vi "MAI-SIM control.vi"() -> ()   [LabVIEW 2021]
uses:
  <vilib>/DAQmx/write.llb/DAQmx Write (Digital Bool 1Line 1Point).vi
  <vilib>/DAQmx/write.llb/DAQmx Write (Analog DBL 1Chan 1Samp).vi
  <vilib>/DAQmx/read.llb/DAQmx Read (Digital Bool 1Line 1Point).vi
  <vilib>/DAQmx/write.llb/DAQmx Write (Analog Wfm 1Chan NSamp).vi
  <vilib>/DAQmx/create/channels.llb/DAQmx Create Channel (DO-Digital Output).vi
  <vilib>/DAQmx/create/channels.llb/DAQmx Create Channel (DI-Digital Input).vi
  <vilib>/Instr/_visa.llb/VISA Configure Serial Port (Instr).vi
  <vilib>/DAQmx/create/channels.llb/DAQmx Create Channel (AO-Voltage-Basic).vi
  <vilib>/DAQmx/miscellaneous.llb/DAQmx Fill In Error Info.vi
  <vilib>/measure/NI_MABase.lvlib
panel:
  out "?":bool=TRUE
  in  "Go live":bool
  in  "stop":bool=TRUE
  in  "Go SIM":bool
  in  "Tab Control":T1(tab)=enum."Voltages"
  in  "Jog Z":bool
  in  "acquire 405":bool
  in  "405 Exp":dbl=150.0
  out "Images needed":dbl=12.0
  in  "5 phases":bool
  in  "Exposure time":dbl=50.0
  in  "interval /s":dbl
  in  "Timepoints":u32=1 min=1 max=1000 step=1
  in  "647":bool
  in  "561":bool
  in  "488":bool
  in  "405":bool
  in  "Steps /um":dbl
  in  "z-slices":dbl=1.0
  in  "acquire 640":bool
  in  "647 Exp":dbl=150.0
  in  "acquire 561":bool=TRUE
  in  "561 Exp":dbl=80.0
  in  "acquire 488":bool
  in  "488 Exp":dbl=40.0
  in  "Live mode":enum32{"Static", "Strobe", "Widefield", "SIM"}(radio)
  in  "Settle time":u32=30
  in  "Optosplit":T2(radio)=enum."rolling SIM"
  out "odd/even indicator":bool=TRUE
  out "Current voltage":dbl=0.95 format="%#_13g"
  in  "Boolean":bool
  in  "Radio Buttons":enum32{"V1", "V2", "V3"}(radio)
  in  "Debug":dbl[](array[numeric])=[0.95, 0.951, 0.952]
  in  "647 voltages":dbl[][](array[numeric])=[[0.95, 2.25, 3.5], [0.951233, 2.25066, 3.50146], [0.952466, 2.25132, 3.50293]]
  in  "561 voltages":dbl[][](array[numeric])=[[0.95, 2.2, 3.5], [0.951, 2.2025, 3.509], [0.952, 2.2056, 3.518]]
  in  "488 voltages":dbl[][](array[numeric])=[[0.95, 2.25, 3.5], [0.95093, 2.25193, 3.50117], [0.95186, 2.25385, 3.50233]]
  in  "405 voltages":dbl[][](array[numeric])=[[1.0, 0.0, 0.0], [0.0, 0.0, 0.0], [0.0, 0.0, 4.0]]
  out "x+y":i32=8
  in  "647 voltages":dbl[][](array[numeric])=[[0.96, 2.2, 3.5], [0.97, 2.2035, 3.5085], [0.975, 2.2045, 3.5118]]
  in  "561 voltages":dbl[][](array[numeric])=[[0.85, 1.91, 3.2], [0.85065, 1.91064, 3.204], [0.85013, 1.91128, 3.208]]
  in  "488 voltages":dbl[][](array[numeric])=[[0.96, 2.2, 3.5], [0.97, 2.2045, 3.51], [0.975, 2.209, 3.52]]
  in  "405 voltages":dbl[][](array[numeric])=[[1.0, 0.0, 0.0], [0.0, 0.0, 0.0], [0.0, 0.0, 4.0]]
  in  "AOTF channel 2":refnum<visa-resource-name>="COM9"
  in  "405 power":dbl(slide)=1.7857142857142856 min=0.0 max=100.0 step=0.05 scale=0.0..100.0
  in  "405 channel":refnum<visa-resource-name>="COM8"
  in  "488 channel":refnum<visa-resource-name>="COM7"
  in  "488 power":dbl(slide)=1.7647058823529411 min=0.0 max=100.0 step=0.05 scale=0.0..100.0
  in  "ASI stage channel":refnum<visa-resource-name>="COM3"
  in  "physical channels":tag="Dev1/ao0"
  in  "expose any":tag="Dev1/port0/line5"
  in  "647 Power":ext(slide)=14.25 scale=0.0..100.0
  in  "405 shutter":tag="Dev1/port0/line8"
  in  "561 shutter":tag="Dev1/port0/line0"
  in  "488 shutter":tag="Dev1/port0/line1"
  in  "Busy in":tag="Dev1/port0/line3"
  in  "Exposure out":tag="Dev1/port0/line2"
  in  "647 channel":refnum<visa-resource-name>="COM5"
  in  "561 power":dbl(slide)=32.142857142857146 min=0.0 max=100.0 step=0.05 scale=0.0..100.0
  in  "Tab Control 2":T3(tab)
  out "Initialisation error":errorcluster
  out "stage error":errorcluster
  out "Camera/galvo error":errorcluster
  out "Laser error":errorcluster
  out "optosplit stage error":errorcluster
  out "resulting string":string="movrel z=0.000000 \r\n"
  out "resulting string 2":string="movrel z=-0.000000 \r\n"
  in  "short delay":dbl=5.0
  in  "long delay":dbl=55.0
  # "Acquire mode"
  # "o"
  # "o"
  # "o"
  # "o"
  # "o"
  # "o"
  # "o"
  # "o"
  # "o"
  # "o"
  # "o"
  # "o"
  # "-60"
  # "0"
  # "60"
  # "-60"
  # "0"
  # "60"
  # "-60"
  # "0"
  # "60"
  # "-60"
  # "0"
  # "60"
  # "0"
  # "2p/3"
  # "4p/3"
  # "o"
  # "o"
  # "o"
  # "o"
  # "o"
  # "o"
  # "o"
  # "o"
  # "o"
  # "o"
  # "o"
  # "o"
  # "-60"
  # "0"
  # "60"
  # "-60"
  # "0"
  # "60"
  # "-60"
  # "0"
  # "60"
  # "-60"
  # "0"
  # "60"
  # "0"
  # "3p/5"
  # "5p/5"
  # "7p/5"
  # "9p/5"
  # "Hardware lines"
  # "Camera lines"
  # "Laser control"
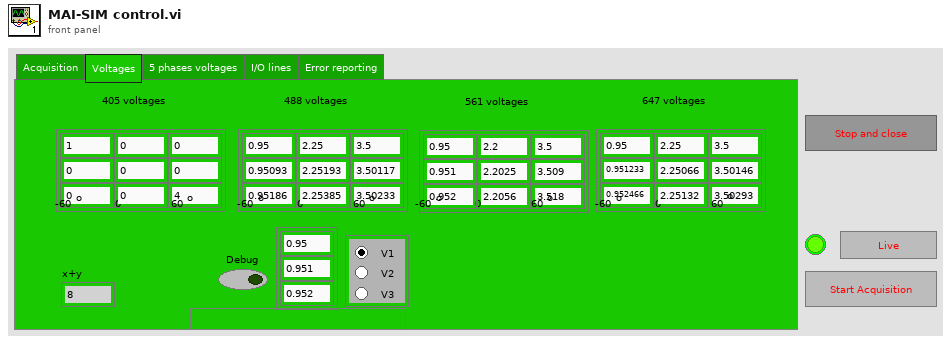
[diagram p1: front panel]
types:
  T1 = enum32{"Acquisition", "Voltages", "5 phases voltages", "I/O lines", "Error reporting"}
  T2 = enum32{"sequential", "optosplit", "fast sequence", "rolling SIM"}
  T3 = enum32{"Page 1", "Page 2", "Page 3", "Page 4", "Page 5"}
  T4 = enum8{"Enabled", "Disabled", "Disabled and Grayed Out"}
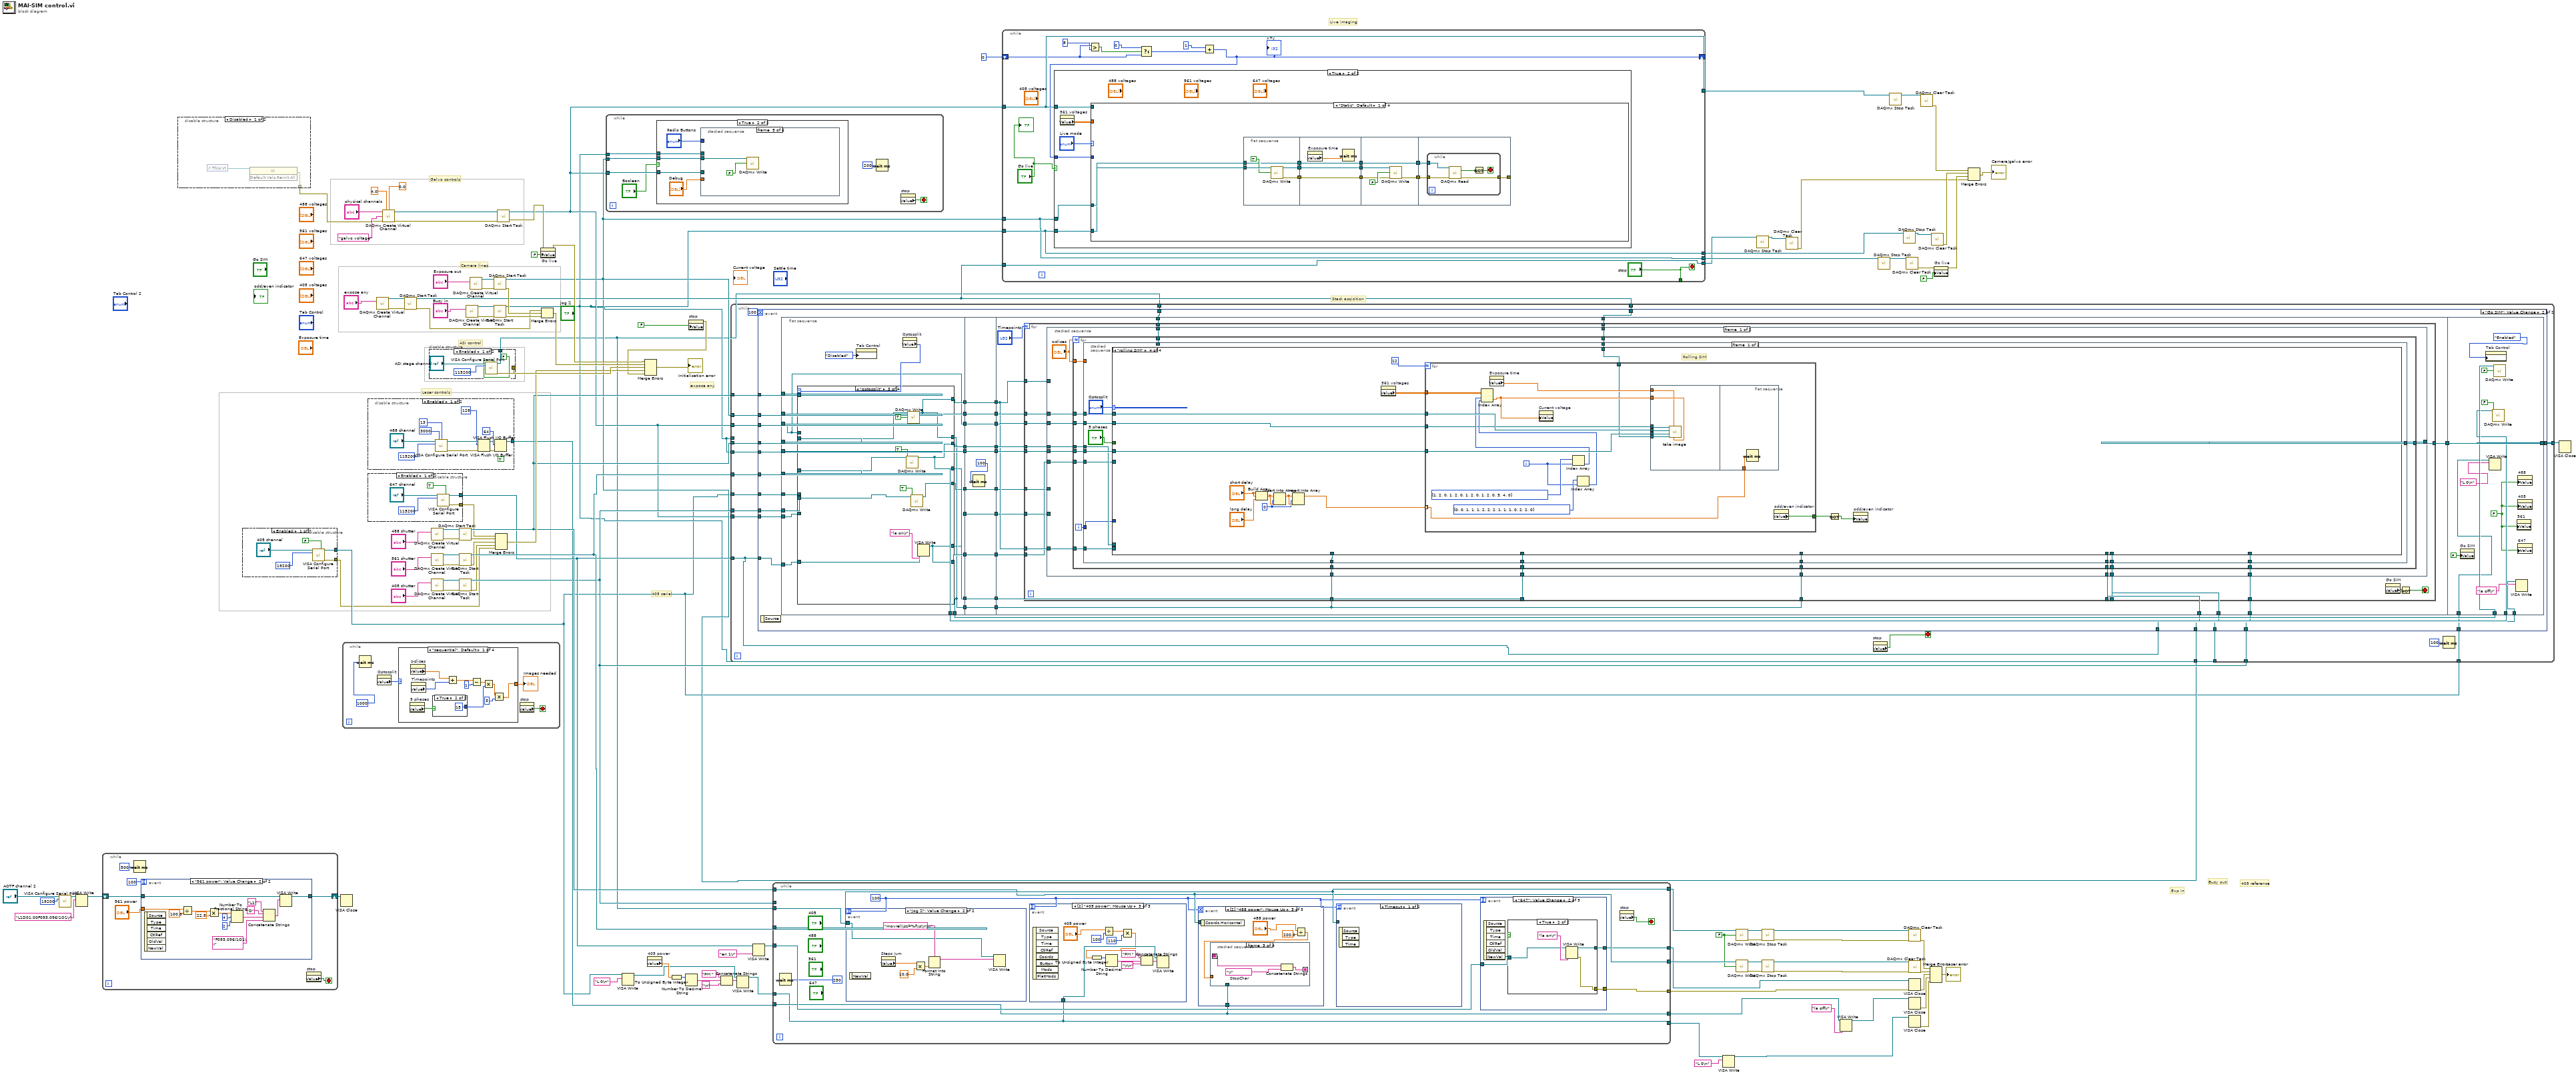
[diagram p0: block diagram]
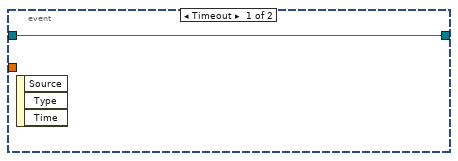
[diagram p2: hidden frame]
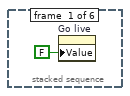
[diagram p7: hidden frame]
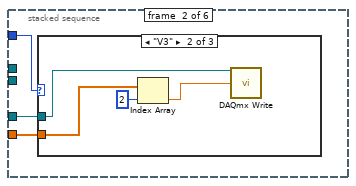
[diagram p8: hidden frame]
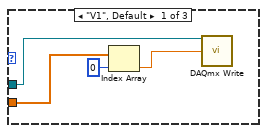
[diagram p9: hidden frame]
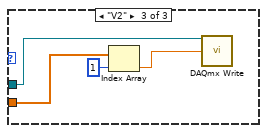
[diagram p10: hidden frame]
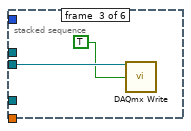
[diagram p11: hidden frame]
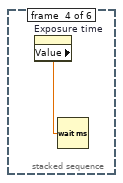
[diagram p12: hidden frame]
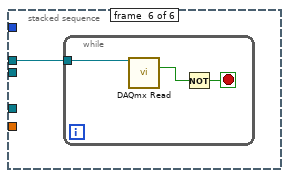
[diagram p13: hidden frame]
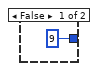
[diagram p15: hidden frame]
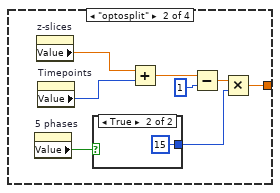
[diagram p16: hidden frame]
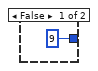
[diagram p17: hidden frame]
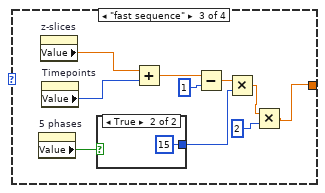
[diagram p18: hidden frame]
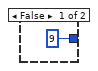
[diagram p19: hidden frame]
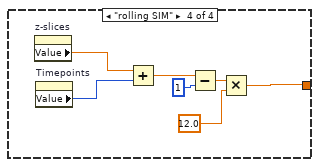
[diagram p20: hidden frame]
diagram:
  w79 = FALSE
  # "405 serial"
  # "expose any"
  # "Busy out"
  # "Exp in"
  # "405 reference"
  # "Stack acqisition"
  # "Live imaging"
  # "Laser controls"
  # "ASI control"
  # "Camera lines"
  # "Galvo controls"
  n1 = call-poly "VISA Configure Serial Port"("VISA resource name"="AOTF channel 2", "baud rate (9600)"=u32 19200) -> ("VISA resource name out"=w2:refnum<visa-resource-name>)  [unwired: 12 in, 1 out]
  n2 = VISA Write(VISA resource name=w2, write buffer="L1D01.00F093.096I1O1\r") -> (VISA resource name out=w1:refnum<visa-resource-name>)  [unwired: 1 in, 2 out]
  n3 = while {
    shift-right: [w116] -> w4
    shift-left: w1 -> [w117]
    stop <- w115 stop-if-true
    n4 = Wait (ms)(milliseconds to wait=500) -> ()  [unwired: 1 out]
    n5 = event shown="[1] \"561 power\": Value Change" {
      selector: _ -> [_ _]
      dyn-events: _ -> [_ _]
      timeout: 100 -> [_ _]
      tunnel: "561 power" -> [_ w132]
      tunnel: w117 -> [w119 w122]
      tunnel: [w119 w121] -> w116
      event Timeout {
        n6 = event-data() -> ()  [unwired: 1 in, 3 out]
      }
      event "561 power": Value Change {
        n7 = event-data() -> ()  [unwired: 1 in, 6 out]
        n8 = Divide(x=w132, y=100.0) -> (x/y=w129:dbl)
        n9 = Multiply(x=w129, y=22.5) -> (x*y=w127:dbl)
        n10 = Number To Fractional String(number=w127, width (-)=4, precision (6)=2) -> (F-format string=w125:string)  [unwired: 1 in]
        n11 = Concatenate Strings("L1", "D", w125, "F093.096I1O1\r") -> (w120:string)
        n12 = VISA Write(VISA resource name=w122, write buffer=w120) -> (VISA resource name out=w121:refnum<visa-resource-name>)  [unwired: 1 in, 2 out]
      }
    }
    n13 = property on="stop" class="Bool (strict)"() -> ("Value"=w115:bool)  [unwired: 2 in, 2 out]
  }
  n14 = disable-structure shown="Disabled" {
    disable-tunnel: [w135 _] -> w26
    frame Disabled {
      n15 = control-ref of="This VI"() -> (w134:refnum<vi>)
      n16 = invoke class="VI" method="Default Vals.Reinit All"(reference=w134) -> (error out=w135:errorcluster)  [unwired: 2 in, 2 out]
    }
    frame Enabled {
    }
  }
  n17 = disable-structure shown="Enabled" {
    disable-tunnel: [w137 _] -> w8
    disable-tunnel: [w136 _] -> w7
    frame Enabled {
      n18 = call-poly "VISA Configure Serial Port"("VISA resource name"="405 channel", "Enable Termination\nChar (T)"=FALSE ("Enable Termination\nChar (T)"), "baud rate (9600)"=u32 19200) -> ("VISA resource name out"=w137:refnum<visa-resource-name>, "error out"=w136:errorcluster)  [unwired: 11 in]
    }
    frame Disabled {
    }
  }
  n19 = VISA Close(VISA resource name=w4) -> ()  [unwired: 1 in, 1 out]
  n20 = while {
    stop <- w143 stop-if-true
    n21 = Wait (ms)(milliseconds to wait=1000) -> ()  [unwired: 1 out]
    n22 = property on="Optosplit" class="RadioBtnsControl (strict)"() -> ("Value"=w142:T2)  [unwired: 2 in, 2 out]
    n23 = case shown="\"sequential\", Default" w142 {
      tunnel: [w145 w162 w167 w180] -> w144
      frame "sequential", Default {
        n24 = property on="5 phases" class="Bool (strict)"() -> ("Value"=w154:bool)  [unwired: 2 in, 2 out]
        n25 = property on="z-slices" class="DigNum (strict)"() -> ("Value"=w152:dbl)  [unwired: 2 in, 2 out]
        n26 = property on="Timepoints" class="DigNum (strict)"() -> ("Value"=w151:u32)  [unwired: 2 in, 2 out]
        n27 = case shown="True" w154 {
          tunnel: [9 15] -> w153
          frame False {
          }
          frame True {
          }
        }
        n28 = Add(x=w152, y=w151) -> (x+y=w149:dbl)
        n29 = Subtract(x=w149, y=1) -> (x-y=w148:dbl)
        n30 = Multiply(x=w148, y=w153) -> (x*y=w147:dbl)
        n31 = Multiply(x=w147, y=3) -> (x*y=w145:dbl)
      }
      frame "optosplit" {
        n32 = property on="5 phases" class="Bool (strict)"() -> ("Value"=w164:bool)  [unwired: 2 in, 2 out]
        n33 = property on="z-slices" class="DigNum (strict)"() -> ("Value"=w161:dbl)  [unwired: 2 in, 2 out]
        n34 = property on="Timepoints" class="DigNum (strict)"() -> ("Value"=w160:u32)  [unwired: 2 in, 2 out]
        n35 = case shown="True" w164 {
          tunnel: [9 15] -> w163
          frame False {
          }
          frame True {
          }
        }
        n36 = Add(x=w161, y=w160) -> (x+y=w158:dbl)
        n37 = Subtract(x=w158, y=1) -> (x-y=w157:dbl)
        n38 = Multiply(x=w157, y=w163) -> (x*y=w162:dbl)
      }
      frame "fast sequence" {
        n39 = property on="5 phases" class="Bool (strict)"() -> ("Value"=w176:bool)  [unwired: 2 in, 2 out]
        n40 = property on="z-slices" class="DigNum (strict)"() -> ("Value"=w174:dbl)  [unwired: 2 in, 2 out]
        n41 = property on="Timepoints" class="DigNum (strict)"() -> ("Value"=w173:u32)  [unwired: 2 in, 2 out]
        n42 = case shown="True" w176 {
          tunnel: [9 15] -> w175
          frame False {
          }
          frame True {
          }
        }
        n43 = Add(x=w174, y=w173) -> (x+y=w171:dbl)
        n44 = Subtract(x=w171, y=1) -> (x-y=w170:dbl)
        n45 = Multiply(x=w170, y=w175) -> (x*y=w169:dbl)
        n46 = Multiply(x=w169, y=2) -> (x*y=w167:dbl)
      }
      frame "rolling SIM" {
        n47 = property on="z-slices" class="DigNum (strict)"() -> ("Value"=w185:dbl)  [unwired: 2 in, 2 out]
        n48 = property on="Timepoints" class="DigNum (strict)"() -> ("Value"=w184:u32)  [unwired: 2 in, 2 out]
        n49 = Add(x=w185, y=w184) -> (x+y=w182:dbl)
        n50 = Subtract(x=w182, y=1) -> (x-y=w181:dbl)
        n51 = Multiply(x=w181, y=12.0) -> (x*y=w180:dbl)
      }
    }
    "Images needed" <- w144
    n52 = property on="stop" class="Bool (strict)"() -> ("Value"=w143:bool)  [unwired: 2 in, 2 out]
  }
  n53 = disable-structure shown="Enabled" {
    disable-tunnel: [w186 _] -> w29
    frame Enabled {
      (unwired) TRUE ("Enable Termination\nChar (T)")
      n54 = call-poly "VISA Configure Serial Port"("VISA resource name"="488 channel", "timeout (10sec)"=u32 3000, "termination char\n(0xA = '\\n' = LF)"=u8 13 ("termination char\n(0xA = '\\n' = LF)"), "baud rate (9600)"=u32 115200) -> ("VISA resource name out"=w196:refnum<visa-resource-name>, "error out"=w195:errorcluster)  [unwired: 5 in, 5 out]
      n55 = VISA Flush I/O Buffer(VISA resource name=w196, mask (16)=u16 128, error in (no error)=w195) -> (VISA resource name out=w192:refnum<visa-resource-name>, error out=w191:errorcluster)
      n56 = VISA Flush I/O Buffer(VISA resource name=w192, mask (16)=u16 64, error in (no error)=w191) -> (VISA resource name out=w186:refnum<visa-resource-name>)  [unwired: 1 out]
    }
    frame Disabled {
    }
  }
  n57 = disable-structure shown="Enabled" {
    disable-tunnel: [w198 _] -> w56
    disable-tunnel: [w197 _] -> w58
    frame Enabled {
      n58 = call-poly "VISA Configure Serial Port"("VISA resource name"="647 channel", "Enable Termination\nChar (T)"=TRUE ("Enable Termination\nChar (T)"), "baud rate (9600)"=u32 115200) -> ("VISA resource name out"=w198:refnum<visa-resource-name>, "error out"=w197:errorcluster)  [unwired: 11 in]
    }
    frame Disabled {
    }
  }
  n59 = call-poly <vilib>:"DAQmx Create Virtual Channel.vi"("lines"="expose any") -> ("task out"=w42:refnum<k21>, "error out"=w41:errorcluster)  [unwired: 13 in]
  n60 = call-poly <vilib>:"DAQmx Create Virtual Channel.vi"("maximum value"=4.0, "minimum value"=0.0, "physical channels"="physical channels", "name to assign"="galvo voltage", "error in"=w26) -> ("task out"=w35:refnum<k21>, "error out"=w34:errorcluster)  [unwired: 9 in]
  n61 = call <vilib>:"DAQmx Start Task.vi"("task/channels in"=w42, "error in"=w41) -> ("task out"=w39:refnum<k21>, "error out"=w40:errorcluster)  [unwired: 12 in]
  n62 = disable-structure shown="Enabled" {
    disable-tunnel: [w204 _] -> w96
    disable-tunnel: [w203 _] -> w25
    frame Enabled {
      n63 = call-poly "VISA Configure Serial Port"("VISA resource name"="ASI stage channel", "Enable Termination\nChar (T)"=FALSE, "baud rate (9600)"=u32 115200) -> ("VISA resource name out"=w203:refnum<visa-resource-name>, "error out"=w204:errorcluster)  [unwired: 11 in]
    }
    frame Disabled {
    }
  }
  n64 = call-poly <vilib>:"DAQmx Create Virtual Channel.vi"("lines"="488 shutter") -> ("task out"=w107:refnum<k21>, "error out"=w108:errorcluster)  [unwired: 13 in]
  n65 = call-poly <vilib>:"DAQmx Create Virtual Channel.vi"("lines"="561 shutter") -> ("task out"=w105:refnum<k21>, "error out"=w106:errorcluster)  [unwired: 13 in]
  n66 = call-poly <vilib>:"DAQmx Create Virtual Channel.vi"("lines"="405 shutter") -> ("task out"=w62:refnum<k21>, "error out"=w63:errorcluster)  [unwired: 13 in]
  n67 = call <vilib>:"DAQmx Start Task.vi"("task/channels in"=w107, "error in"=w108) -> ("task out"=w91:refnum<k21>, "error out"=w100:errorcluster)  [unwired: 12 in]
  n68 = call <vilib>:"DAQmx Start Task.vi"("task/channels in"=w105, "error in"=w106) -> ("task out"=w92:refnum<k21>, "error out"=w99:errorcluster)  [unwired: 12 in]
  n69 = call <vilib>:"DAQmx Start Task.vi"("task/channels in"=w62, "error in"=w63) -> ("task out"=w54:refnum<k21>, "error out"=w30:errorcluster)  [unwired: 12 in]
  n70 = call-poly <vilib>:"DAQmx Create Virtual Channel.vi"("lines"="Busy in") -> ("task out"=w109:refnum<k21>, "error out"=w110:errorcluster)  [unwired: 13 in]
  n71 = call-poly <vilib>:"DAQmx Create Virtual Channel.vi"("lines"="Exposure out") -> ("task out"=w112:refnum<k21>, "error out"=w111:errorcluster)  [unwired: 13 in]
  n72 = call <vilib>:"DAQmx Start Task.vi"("task/channels in"=w112, "error in"=w111) -> ("task out"=w32:refnum<k21>, "error out"=w98:errorcluster)  [unwired: 12 in]
  n73 = call <vilib>:"DAQmx Start Task.vi"("task/channels in"=w109, "error in"=w110) -> ("task out"=w27:refnum<k21>, "error out"=w97:errorcluster)  [unwired: 12 in]
  n74 = Merge Errors(w58, w100, w99, w30, w7) -> (w94:errorcluster)
  n75 = call <vilib>:"DAQmx Start Task.vi"("task/channels in"=w35, "error in"=w34) -> ("task out"=w31:refnum<k21>, "error out"=w52:errorcluster)  [unwired: 12 in]
  n76 = property on="Go live" class="Bool (strict)"(error in=w52, "Value"=FALSE) -> (error out=w51:errorcluster)  [unwired: 1 in, 1 out]
  n77 = Merge Errors(w40, w98, w97) -> (w95:errorcluster)
  n78 = while {
    tunnel: w32 -> [w211]
    tunnel: w27 -> [w210]
    tunnel: w31 -> [w209]
    stop <- w212 stop-if-true
    n79 = case shown="True" "Boolean" {
      tunnel: w211 -> [_ w217]
      tunnel: w210 -> [_ w216]
      tunnel: w209 -> [_ w215]
      frame False {
      }
      frame True {
        n80 = stacked-sequence {
          tunnel: w217 -> [_ _ w235 _ w237 _]
          tunnel: w216 -> [_ _ _ _ _ w239]
          tunnel: "Radio Buttons" -> [_ w221 _ _ _ _]
          tunnel: "Debug" -> [_ w220 _ _ _ _]
          tunnel: w215 -> [_ w219 _ _ _ _]
          frame #0 {
            n81 = property on="Go live" class="Bool (strict)"("Value"=FALSE ("Go live")) -> ()  [unwired: 2 in, 2 out]
          }
          frame #1 {
            n82 = case shown="\"V3\"" w221 {
              tunnel: w220 -> [w224 w228 w232]
              tunnel: w219 -> [w225 w229 w233]
              frame "V1", Default {
                n83 = Index Array(array=w224, index=0) -> (element=w223:dbl)
                n84 = call-poly <vilib>:"DAQmx Write.vi"("task/channels in"=w225, "data"=w223) -> ()  [unwired: 11 in, 3 out]
              }
              frame "V3" {
                n85 = Index Array(array=w228, index=2) -> (element=w227:dbl)
                n86 = call-poly <vilib>:"DAQmx Write.vi"("task/channels in"=w229, "data"=w227) -> ()  [unwired: 11 in, 3 out]
              }
              frame "V2" {
                n87 = Index Array(array=w232, index=1) -> (element=w231:dbl)
                n88 = call-poly <vilib>:"DAQmx Write.vi"("task/channels in"=w233, "data"=w231) -> ()  [unwired: 11 in, 3 out]
              }
            }
          }
          frame #2 {
            n89 = call-poly <vilib>:"DAQmx Write.vi"("task/channels in"=w235, "data"=TRUE) -> ()  [unwired: 11 in, 3 out]
          }
          frame #3 {
            n90 = property on="Exposure time" class="DigNum (strict)"() -> ("Value"=w236:dbl)  [unwired: 2 in, 2 out]
            n91 = Wait (ms)(milliseconds to wait=w236) -> ()  [unwired: 1 out]
          }
          frame #4 {
            n92 = call-poly <vilib>:"DAQmx Write.vi"("task/channels in"=w237, "data"=FALSE) -> ()  [unwired: 11 in, 3 out]
          }
          frame #5 {
            n93 = while {
              tunnel: w239 -> [w240]
              stop <- w242 stop-if-true
              n94 = call-poly <vilib>:"DAQmx Read.vi"("task/channels in"=w240) -> ("data"=w241:bool)  [unwired: 12 in, 2 out]
              n95 = Not(x=w241) -> (.not. x?=w242:bool)
            }
          }
        }
      }
    }
    n96 = Wait (ms)(milliseconds to wait=u32 200) -> ()  [unwired: 1 out]
    n97 = property on="stop" class="Bool (strict)"() -> ("Value"=w212:bool)  [unwired: 2 in, 2 out]
  }
  n98 = VISA Write(VISA resource name=w8, write buffer="L 0\n" ("format string")) -> (VISA resource name out=w17:refnum<visa-resource-name>)  [unwired: 1 in, 2 out]
  n99 = property on="405 power" class="Slide (strict)"() -> ("Value"=w18:dbl)  [unwired: 2 in, 2 out]
  n100 = To Unsigned Byte Integer(number=w18) -> (unsigned 8bit integer=w19:u8)
  n101 = Number To Decimal String(number=w19) -> (decimal integer string=w21:string)  [unwired: 1 in]
  n102 = property on="stop" class="Bool (strict)"("Value"=FALSE) -> (error out=w65:errorcluster)  [unwired: 2 in, 1 out]
  n103 = Merge Errors(w51, w95, w96, w94, w65) -> (→"Initialisation error":errorcluster)
  n104 = Concatenate Strings("PM ", w21, "\n") -> (w23:string)
  n105 = while {
    tunnel: w32 -> [w261]
    tunnel: w27 -> [w260]
    tunnel: w31 -> [w259]
    tunnel: w91 -> [w258]
    tunnel: w92 -> [w257]
    tunnel: w91 -> [w256]
    tunnel: w25 -> [w254]
    tunnel: [w253] -> w67
    tunnel: w27 -> [_]
    tunnel: w56 -> [w251]
    tunnel: w54 -> [w252]
    tunnel: w54 -> [w250]
    tunnel: w32 -> [w249]
    tunnel: w27 -> [w248]
    tunnel: w31 -> [w247]
    tunnel: w39 -> [w246]
    tunnel: w8 -> [w244]
    tunnel: w8 -> [w243]
    stop <- w255 stop-if-true
    n106 = event shown="[1] \"Go SIM\": Value Change" {
      selector: _ -> [_ _]
      dyn-events: _ -> [_ _]
      timeout: 100 -> [_ _]
      tunnel: w261 -> [_ w304]
      tunnel: w260 -> [_ w303]
      tunnel: w259 -> [_ w302]
      tunnel: w258 -> [_ w301]
      tunnel: w257 -> [_ w300]
      tunnel: w256 -> [_ w299]
      tunnel: w254 -> [w263 w298]
      tunnel: [w263 w297] -> w253
      tunnel: w251 -> [_ w293]
      tunnel: w252 -> [_ w292]
      tunnel: w251 -> [_ w291]
      tunnel: w250 -> [_ w290]
      tunnel: w249 -> [_ w289]
      tunnel: w248 -> [_ w288]
      tunnel: w247 -> [_ w287]
      tunnel: w246 -> [_ w266]
      tunnel: w244 -> [_ w265]
      tunnel: w243 -> [_ w264]
      event Timeout {
        n107 = event-data() -> ()  [unwired: 1 in, 3 out]
      }
      event "Go SIM": Value Change {
        n108 = event-data() -> ()  [unwired: 1 in, 1 out]
        n109 = flat-sequence {
          tunnel: [w323] -> w286
          tunnel: w304 -> [w323]
          tunnel: [w322] -> w284
          tunnel: w303 -> [w322]
          tunnel: [w307] -> w282
          tunnel: w302 -> [w307]
          tunnel: w301 -> [w320]
          tunnel: w300 -> [w319]
          tunnel: w299 -> [w318]
          tunnel: [w317] -> w280
          tunnel: [w316] -> w278
          tunnel: [w312] -> w294
          tunnel: [w311] -> w295
          tunnel: w293 -> [w315]
          tunnel: w292 -> [w314]
          tunnel: [w313] -> w276
          tunnel: [w312] -> w274
          tunnel: [w311] -> w272
          tunnel: w287 -> [w310]
          tunnel: [w309] -> w269
          tunnel: [w308] -> w267
          tunnel: w265 -> [w305]
          tunnel: w286 -> [w417]
          tunnel: [w417] -> w285
          tunnel: w284 -> [w416]
          tunnel: [w416] -> w283
          tunnel: w282 -> [w415]
          tunnel: [w415] -> w281
          tunnel: w280 -> [w414]
          tunnel: [w414] -> w279
          tunnel: w278 -> [w413]
          tunnel: [w413] -> w277
          tunnel: w276 -> [w412]
          tunnel: [w412] -> w275
          tunnel: w274 -> [w411]
          tunnel: [w411] -> w273
          tunnel: w272 -> [w410]
          tunnel: [w410] -> w271
          tunnel: [w408] -> w270
          tunnel: w269 -> [w408]
          tunnel: [w407] -> w268
          tunnel: w267 -> [w407]
          tunnel: w285 -> [w434]
          tunnel: w283 -> [w433]
          tunnel: w281 -> [w432]
          tunnel: w279 -> [w431]
          tunnel: w277 -> [w422]
          tunnel: w298 -> [w430]
          tunnel: [w429] -> w296
          tunnel: w275 -> [w428]
          tunnel: w273 -> [w426]
          tunnel: w271 -> [w427]
          tunnel: w290 -> [w425]
          tunnel: w289 -> [w424]
          tunnel: w288 -> [w423]
          tunnel: w270 -> [w421]
          tunnel: w268 -> [w420]
          tunnel: w266 -> [w419]
          tunnel: [w1232] -> w297
          tunnel: w296 -> [w1232]
          tunnel: w295 -> [w1228]
          tunnel: w294 -> [w1229]
          tunnel: w291 -> [w1226]
          tunnel: w264 -> [w1222]
          frame #0 {
            n110 = property on="Tab Control" class="TabCtl (strict)"("DisabledEnum"=T4."Disabled" ("Disabled")) -> ()  [unwired: 2 in, 2 out]
            n111 = property on="Optosplit" class="RadioBtnsControl (strict)"() -> ("Value"=w321:T2)  [unwired: 2 in, 2 out]
            n112 = case shown="\"optosplit\"" w321 {
              tunnel: w320 -> [_ _ _ _]
              tunnel: w319 -> [w334 w356 w375 w394]
              tunnel: w318 -> [w335 w357 w377 w396]
              tunnel: [w333 w355 w374 w393] -> w317
              tunnel: [w332 w354 w376 w395] -> w316
              tunnel: [w333 w355 w374 w393] -> w311
              tunnel: [w332 w354 w376 w395] -> w312
              tunnel: w315 -> [w327 w349 w372 w392]
              tunnel: w314 -> [w330 w352 w370 w382]
              tunnel: [w324 w346 w368 w391] -> w313
              tunnel: [w328 w350 w369 w382] -> w309
              tunnel: w310 -> [w325 w348 _ _]
              tunnel: [w324 w346 w368 w391] -> w308
              tunnel: w307 -> [_ _ _ w383]
              tunnel: w305 -> [_ _ _ w380]
              frame "sequential", Default {
                n113 = property on="odd/even indicator" class="Bool (strict)"() -> ("Value"=w326:bool)  [unwired: 2 in, 2 out]
                n114 = case shown="True" w326 {
                  tunnel: w325 -> [w341 w345]
                  frame False {
                    w339 = 2
                    n115 = property on="647 voltages" class="Arr (strict)"() -> ("Value"=w340:dbl[][])  [unwired: 2 in, 2 out]
                    n116 = Index Array(array=w340, index (row)=w339, index (col)=w339) -> (element=w338:dbl)
                    n117 = call-poly <vilib>:"DAQmx Write.vi"("task/channels in"=w341, "data"=w338) -> ()  [unwired: 11 in, 3 out]
                  }
                  frame True {
                    w343 = 0
                    n118 = property on="561 voltages" class="Arr (strict)"() -> ("Value"=w344:dbl[][])  [unwired: 2 in, 2 out]
                    n119 = Index Array(array=w344, index (row)=w343, index (col)=w343) -> (element=w342:dbl)
                    n120 = call-poly <vilib>:"DAQmx Write.vi"("task/channels in"=w345, "data"=w342) -> ()  [unwired: 11 in, 3 out]
                  }
                }
                n121 = call-poly <vilib>:"DAQmx Write.vi"("task/channels in"=w330, "data"=FALSE) -> ("task out"=w328:refnum<k21>)  [unwired: 11 in, 2 out]
                n122 = call-poly <vilib>:"DAQmx Write.vi"("task/channels in"=w334, "data"=FALSE) -> ("task out"=w333:refnum<k21>)  [unwired: 11 in, 2 out]
                n123 = call-poly <vilib>:"DAQmx Write.vi"("task/channels in"=w335, "data"=FALSE) -> ("task out"=w332:refnum<k21>)  [unwired: 11 in, 2 out]
                n124 = VISA Write(VISA resource name=w327, write buffer="la off\r" ("format string")) -> (VISA resource name out=w324:refnum<visa-resource-name>)  [unwired: 1 in, 2 out]
              }
              frame "fast sequence" {
                n125 = property on="odd/even indicator" class="Bool (strict)"() -> ("Value"=w347:bool)  [unwired: 2 in, 2 out]
                n126 = case shown="True" w347 {
                  tunnel: w348 -> [w363 w367]
                  frame False {
                    w361 = 2
                    n127 = property on="647 voltages" class="Arr (strict)"() -> ("Value"=w362:dbl[][])  [unwired: 2 in, 2 out]
                    n128 = Index Array(array=w362, index (row)=w361, index (col)=w361) -> (element=w360:dbl)
                    n129 = call-poly <vilib>:"DAQmx Write.vi"("task/channels in"=w363, "data"=w360) -> ()  [unwired: 11 in, 3 out]
                  }
                  frame True {
                    w365 = 0
                    n130 = property on="647 voltages" class="Arr (strict)"() -> ("Value"=w366:dbl[][])  [unwired: 2 in, 2 out]
                    n131 = Index Array(array=w366, index (row)=w365, index (col)=w365) -> (element=w364:dbl)
                    n132 = call-poly <vilib>:"DAQmx Write.vi"("task/channels in"=w367, "data"=w364) -> ()  [unwired: 11 in, 3 out]
                  }
                }
                n133 = call-poly <vilib>:"DAQmx Write.vi"("task/channels in"=w352, "data"=FALSE) -> ("task out"=w350:refnum<k21>)  [unwired: 11 in, 2 out]
                n134 = call-poly <vilib>:"DAQmx Write.vi"("task/channels in"=w356, "data"=FALSE) -> ("task out"=w355:refnum<k21>)  [unwired: 11 in, 2 out]
                n135 = call-poly <vilib>:"DAQmx Write.vi"("task/channels in"=w357, "data"=FALSE) -> ("task out"=w354:refnum<k21>)  [unwired: 11 in, 2 out]
                n136 = VISA Write(VISA resource name=w349, write buffer="la off\r" ("format string")) -> (VISA resource name out=w346:refnum<visa-resource-name>)  [unwired: 1 in, 2 out]
              }
              frame "optosplit" {
                n137 = call-poly <vilib>:"DAQmx Write.vi"("task/channels in"=w375, "data"=TRUE) -> ("task out"=w374:refnum<k21>)  [unwired: 11 in, 2 out]
                n138 = call-poly <vilib>:"DAQmx Write.vi"("task/channels in"=w377, "data"=TRUE) -> ("task out"=w376:refnum<k21>)  [unwired: 11 in, 2 out]
                n139 = call-poly <vilib>:"DAQmx Write.vi"("task/channels in"=w370, "data"=TRUE) -> ("task out"=w369:refnum<k21>)  [unwired: 11 in, 2 out]
                n140 = VISA Write(VISA resource name=w372, write buffer="la on\r" ("format string")) -> (VISA resource name out=w368:refnum<visa-resource-name>)  [unwired: 1 in, 2 out]
              }
              frame "rolling SIM" {
                w387 = 0
                n141 = property on="561 voltages" class="Arr (strict)"() -> ("Value"=w388:dbl[][])  [unwired: 2 in, 2 out]
                n142 = property on="acquire 640" class="Bool (strict)"() -> ("Value"=w384:bool)  [unwired: 2 in, 2 out]
                n143 = property on="z-slices" class="DigNum (strict)"("Value"=1) -> ()  [unwired: 2 in, 2 out]
                n144 = property on="acquire 488" class="Bool (strict)"() -> ("Value"=w386:bool)  [unwired: 2 in, 2 out]
                n145 = Index Array(array=w388, index (row)=w387, index (col)=w387) -> (element=w389:dbl)
                n146 = property on="acquire 561" class="Bool (strict)"() -> ("Value"=w385:bool)  [unwired: 2 in, 2 out]
                n147 = property on="acquire 405" class="Bool (strict)"() -> ("Value"=w381:bool)  [unwired: 2 in, 2 out]
                n148 = call-poly <vilib>:"DAQmx Write.vi"("task/channels in"=w383, "data"=w389) -> ()  [unwired: 11 in, 3 out]
                n149 = case shown="False" w381 {
                  tunnel: w380 -> [w397 w399]
                  frame False {
                    n150 = VISA Write(VISA resource name=w397, write buffer="L 0\n" ("format string")) -> ()  [unwired: 1 in, 3 out]
                  }
                  frame True {
                    n151 = VISA Write(VISA resource name=w399, write buffer="L 1\n" ("format string")) -> ()  [unwired: 1 in, 3 out]
                  }
                }
                n152 = case shown="True" w384 {
                  tunnel: w392 -> [w402 w405]
                  tunnel: [w401 w404] -> w391
                  frame False {
                    n153 = VISA Write(VISA resource name=w402, write buffer="la off\r" ("format string")) -> (VISA resource name out=w401:refnum<visa-resource-name>)  [unwired: 1 in, 2 out]
                  }
                  frame True {
                    n154 = VISA Write(VISA resource name=w405, write buffer="la on\r" ("format string")) -> (VISA resource name out=w404:refnum<visa-resource-name>)  [unwired: 1 in, 2 out]
                  }
                }
                n155 = call-poly <vilib>:"DAQmx Write.vi"("task/channels in"=w394, "data"=w385) -> ("task out"=w393:refnum<k21>)  [unwired: 11 in, 2 out]
                n156 = call-poly <vilib>:"DAQmx Write.vi"("task/channels in"=w396, "data"=w386) -> ("task out"=w395:refnum<k21>)  [unwired: 11 in, 2 out]
              }
            }
          }
          frame #1 {
            n157 = Wait (ms)(milliseconds to wait=100) -> ()  [unwired: 1 out]
          }
          frame #2 {
            n158 = for {
              N: "Timepoints" -> [_]
              tunnel: w434 -> [w454]
              tunnel: w433 -> [w453]
              tunnel: w432 -> [w452]
              tunnel: w431 -> [w451]
              tunnel: w422 -> [w450]
              tunnel: w430 -> [w449]
              tunnel: [w448] -> w429
              tunnel: w428 -> [w447]
              tunnel: w427 -> [w446]
              tunnel: w426 -> [w445]
              tunnel: w426 -> [w444]
              tunnel: w425 -> [w443]
              tunnel: w424 -> [w442]
              tunnel: w423 -> [w441]
              tunnel: w422 -> [w440]
              tunnel: w421 -> [w439]
              tunnel: w420 -> [w438]
              tunnel: w419 -> [w437]
              stop <- w435 stop-if-true
              n159 = stacked-sequence {
                tunnel: w454 -> [w470 _]
                tunnel: w453 -> [w469 _]
                tunnel: w452 -> [w468 _]
                tunnel: w451 -> [w467 w1134]
                tunnel: w450 -> [w466 _]
                tunnel: w449 -> [w465 w1136]
                tunnel: [w464 _] -> w448
                tunnel: w447 -> [w463 _]
                tunnel: w446 -> [w462 _]
                tunnel: w445 -> [w461 _]
                tunnel: w444 -> [w460 _]
                tunnel: w443 -> [w459 _]
                tunnel: w442 -> [w458 _]
                tunnel: w441 -> [w457 _]
                tunnel: w440 -> [_ w1135]
                tunnel: w439 -> [_ w1133]
                tunnel: w438 -> [_ w1132]
                tunnel: w437 -> [w455 _]
                frame #0 {
                  n160 = for {
                    N: "z-slices" -> [_]
                    tunnel: w470 -> [w487]
                    tunnel: w469 -> [w486]
                    tunnel: w468 -> [w485]
                    tunnel: w467 -> [w484]
                    tunnel: w466 -> [w483]
                    tunnel: w465 -> [w482]
                    tunnel: [w481] -> w464
                    tunnel: w463 -> [w480]
                    tunnel: w462 -> [w479]
                    tunnel: w461 -> [w478]
                    tunnel: w460 -> [w477]
                    tunnel: w459 -> [w476]
                    tunnel: w458 -> [w475]
                    tunnel: w457 -> [w474]
                    tunnel: "z-slices" -> [w472]
                    tunnel: w455 -> [w471]
                    i -> [w473]
                    n161 = stacked-sequence {
                      tunnel: w487 -> [w502 _]
                      tunnel: w486 -> [w501 _]
                      tunnel: w485 -> [w500 _]
                      tunnel: w484 -> [w499 _]
                      tunnel: w483 -> [w498 _]
                      tunnel: w482 -> [_ w1104]
                      tunnel: [_ w1103] -> w481
                      tunnel: w480 -> [w496 _]
                      tunnel: w479 -> [w495 _]
                      tunnel: w478 -> [w494 _]
                      tunnel: w477 -> [w493 _]
                      tunnel: w476 -> [w492 _]
                      tunnel: w475 -> [w491 _]
                      tunnel: w474 -> [w490 _]
                      tunnel: w473 -> [w489 _]
                      tunnel: w472 -> [_ w1099]
                      tunnel: w471 -> [w488 _]
                      frame #0 {
                        n162 = case shown="\"rolling SIM\"" "Optosplit" {
                          tunnel: w502 -> [w525 w848 w977 w1074]
                          tunnel: w501 -> [w524 w847 w976 w1073]
                          tunnel: w500 -> [w507 w843 w975 w1067]
                          tunnel: w499 -> [w514 _ _ _]
                          tunnel: w498 -> [w513 _ _ _]
                          tunnel: "5 phases" -> [_ _ w974 _]
                          tunnel: w496 -> [w512 w842 _ _]
                          tunnel: w495 -> [w511 w841 _ _]
                          tunnel: w494 -> [w510 _ _ _]
                          tunnel: w493 -> [_ w836 _ _]
                          tunnel: w492 -> [w509 w835 _ _]
                          tunnel: w491 -> [w506 _ _ _]
                          tunnel: w490 -> [w505 _ _ _]
                          tunnel: w489 -> [_ _ _ _]
                          tunnel: w488 -> [w504 w834 w973 w1068]
                          frame "sequential", Default {
                            # "Without optosplit"
                            n163 = case shown="True" "acquire 640" {
                              tunnel: w525 -> [w753 w763]
                              tunnel: w524 -> [w751 w762]
                              tunnel: w507 -> [w752 w756]
                              tunnel: [w753 w760] -> w520
                              tunnel: [w752 w761] -> w521
                              tunnel: [w751 w759] -> w522
                              tunnel: w512 -> [_ w755]
                              tunnel: w504 -> [_ w754]
                              frame False {
                              }
                              frame True {
                                n164 = property on="647 voltages" class="Arr (strict)"() -> ("Value"=w757:dbl[][])  [unwired: 2 in, 2 out]
                                n165 = stacked-sequence {
                                seq-local: [_ w777 _ _] -> [_ _ w797 _]
                                seq-local: [_ w776 _ _] -> [_ _ w796 _]
                                seq-local: [_ w775 _ _] -> [_ _ w795 _]
                                seq-local: [_ w774 _ _] -> [_ _ w791 _]
                                seq-local: [_ w773 _ _] -> [_ _ w790 _]
                                tunnel: w763 -> [_ w777 _ _]
                                tunnel: w756 -> [_ w776 _ _]
                                tunnel: w762 -> [_ w775 _ _]
                                tunnel: w757 -> [_ w774 _ _]
                                tunnel: "647 Exp" -> [_ w773 _ _]
                                tunnel: [_ _ w794 _] -> w761
                                tunnel: [_ _ w793 _] -> w760
                                tunnel: [_ _ w792 _] -> w759
                                tunnel: w757 -> [_ w772 _ _]
                                tunnel: w756 -> [_ w771 _ _]
                                tunnel: w755 -> [w764 _ _ w831]
                                tunnel: w754 -> [_ _ w788 _]
                                frame #0 {
                                n166 = stacked-sequence {
                                tunnel: w764 -> [w765 _]
                                frame #0 {
                                n167 = VISA Write(VISA resource name=w765, write buffer="la on\r" ("format string")) -> ()  [unwired: 1 in, 3 out]
                                }
                                frame #1 {
                                n168 = Wait (ms)(milliseconds to wait=100) -> ()  [unwired: 1 out]
                                }
                                }
                                }
                                frame #1 {
                                n169 = property on="odd/even indicator" class="Bool (strict)"() -> ("Value"=w768:bool)  [unwired: 2 in, 2 out]
                                n170 = case shown="False" w768 {
                                tunnel: [2 0] -> w770
                                tunnel: [2 0] -> w769
                                frame False {
                                }
                                frame True {
                                }
                                }
                                n171 = flat-sequence {
                                tunnel: [w785] -> _
                                tunnel: w772 -> [w787]
                                tunnel: w771 -> [w785]
                                tunnel: [w786] -> _
                                tunnel: w770 -> [w783]
                                tunnel: w769 -> [w782]
                                frame #0 {
                                n172 = Index Array(array=w787, index (row)=w783, index (col)=w782) -> (element=w784:dbl)
                                n173 = call-poly <vilib>:"DAQmx Write.vi"("task/channels in"=w785, "data"=w784) -> ("task out"=w786:refnum<k21>)  [unwired: 11 in, 2 out]
                                }
                                }
                                }
                                frame #2 {
                                n174 = for {
                                N: 9 -> [_]
                                tunnel: w791 -> [w809]
                                tunnel: w797 -> [w806]
                                tunnel: w796 -> [w807]
                                tunnel: w795 -> [w805]
                                tunnel: w790 -> [w808]
                                tunnel: [w807] -> w794
                                tunnel: [w806] -> w793
                                tunnel: [w805] -> w792
                                tunnel: w788 -> [w798]
                                i -> [w801]
                                n175 = property on="odd/even indicator" class="Bool (strict)"() -> ("Value"=w799:bool)  [unwired: 2 in, 2 out]
                                n176 = case shown="True" w799 {
                                tunnel: [i32[] [1, 0, 2, 1, 0, 2, 1, 0, 0, 0, 1, 2, 3, 4, 0] i32[] [1, 2, 0, 1, 2, 0, 1, 2, 2, 0, 1, 2, 3, 4, 0]] -> w804
                                tunnel: [i32[] [2, 2, 1, 1, 1, 0, 0, 0, 0, 2, 2, 2, 2, 2, 0] i32[] [0, 0, 1, 1, 1, 2, 2, 2, 2, 2, 2, 2, 2, 2, 0]] -> w803
                                frame False {
                                }
                                frame True {
                                }
                                }
                                n177 = Index Array(array=w804, index=w801) -> (element=w802:i32)
                                n178 = flat-sequence {
                                tunnel: w809 -> [w818]
                                tunnel: w808 -> [w822]
                                tunnel: w807 -> [w821]
                                tunnel: w806 -> [w820]
                                tunnel: w805 -> [w819]
                                tunnel: w800 -> [w816]
                                tunnel: w802 -> [w815]
                                tunnel: w798 -> [w814]
                                frame #0 {
                                n179 = Index Array(array=w818, index (row)=w815, index (col)=w816) -> (element=w817:dbl)
                                n180 = call "take image.vi"("Voltage"=w817, "Exposure time"=w822, "expose any"=w814, "Busy out"=w819, "Exp In"=w820, "Galvo"=w821) -> ()  [unwired: 6 in]
                                }
                                frame #1 {
                                n181 = property on="Settle time" class="DigNum (strict)"() -> ("Value"=w823:u32)  [unwired: 2 in, 2 out]
                                n182 = Wait (ms)(milliseconds to wait=w823) -> ()  [unwired: 1 out]
                                }
                                }
                                n183 = Index Array(array=w803, index=w801) -> (element=w800:i32)
                                }
                                }
                                frame #3 {
                                n184 = property on="acquire 488" class="Bool (strict)"() -> ("Value"=w827:bool)  [unwired: 2 in, 2 out]
                                n185 = property on="acquire 405" class="Bool (strict)"() -> ("Value"=w826:bool)  [unwired: 2 in, 2 out]
                                n186 = property on="acquire 561" class="Bool (strict)"() -> ("Value"=w828:bool)  [unwired: 2 in, 2 out]
                                n187 = property on="odd/even indicator" class="Bool (strict)"() -> ("Value"=w829:bool)  [unwired: 2 in, 2 out]
                                n188 = Or(x=w828, y=w827) -> (x .or. y?=w825:bool)
                                n189 = Not(x=w829) -> (.not. x?=w830:bool)
                                n190 = Or(x=w825, y=w826) -> (x .or. y?=w824:bool)
                                n191 = case shown="True" w824 {
                                tunnel: w831 -> [_ w832]
                                frame False {
                                }
                                frame True {
                                n192 = VISA Write(VISA resource name=w832, write buffer="la off\r" ("format string")) -> ()  [unwired: 1 in, 3 out]
                                }
                                }
                                n193 = property on="odd/even indicator" class="Bool (strict)"("Value"=w830) -> ()  [unwired: 2 in, 2 out]
                                }
                                }
                              }
                            }
                            n194 = case shown="True" "acquire 561" {
                              tunnel: w522 -> [w670 w681]
                              tunnel: w521 -> [w671 w682]
                              tunnel: [w669 w679] -> w518
                              tunnel: [w671 w680] -> w517
                              tunnel: [w670 w678] -> w516
                              tunnel: w520 -> [w669 w677]
                              tunnel: w514 -> [_ _]
                              tunnel: w507 -> [_ w674]
                              tunnel: w511 -> [_ w673]
                              tunnel: w504 -> [_ w672]
                              frame False {
                              }
                              frame True {
                                n195 = property on="561 voltages" class="Arr (strict)"() -> ("Value"=w675:dbl[][])  [unwired: 2 in, 2 out]
                                n196 = stacked-sequence {
                                seq-local: [_ w692 _ _] -> [_ _ w714 _]
                                seq-local: [_ w691 _ _] -> [_ _ w713 _]
                                seq-local: [_ w690 _ _] -> [_ _ w709 _]
                                seq-local: [_ w689 _ _] -> [_ _ w707 _]
                                seq-local: [_ w688 _ _] -> [_ _ w706 _]
                                tunnel: w682 -> [_ w692 _ _]
                                tunnel: w681 -> [_ w691 _ _]
                                tunnel: w677 -> [_ w690 _ _]
                                tunnel: w675 -> [_ w689 _ _]
                                tunnel: "561 Exp" -> [_ w688 _ _]
                                tunnel: [_ _ w712 _] -> w680
                                tunnel: [_ _ w711 _] -> w679
                                tunnel: [_ _ w710 _] -> w678
                                tunnel: w675 -> [_ w686 _ _]
                                tunnel: w674 -> [_ w685 _ _]
                                tunnel: w673 -> [w684 _ _ w748]
                                tunnel: w672 -> [_ _ w705 _]
                                frame #0 {
                                n197 = call-poly <vilib>:"DAQmx Write.vi"("task/channels in"=w684, "data"=TRUE) -> ()  [unwired: 11 in, 3 out]
                                }
                                frame #1 {
                                n198 = flat-sequence {
                                tunnel: w686 -> [w696]
                                tunnel: [w695] -> w687
                                tunnel: w685 -> [w694]
                                tunnel: [w704] -> _
                                tunnel: w687 -> [w704]
                                frame #0 {
                                n199 = property on="odd/even indicator" class="Bool (strict)"() -> ("Value"=w693:bool)  [unwired: 2 in, 2 out]
                                n200 = case shown="True" w693 {
                                tunnel: [2 0] -> w699
                                tunnel: [2 0] -> w698
                                frame False {
                                }
                                frame True {
                                }
                                }
                                n201 = Index Array(array=w696, index (row)=w699, index (col)=w698) -> (element=w697:dbl)
                                n202 = call-poly <vilib>:"DAQmx Write.vi"("task/channels in"=w694, "data"=w697) -> ("task out"=w695:refnum<k21>)  [unwired: 11 in, 2 out]
                                }
                                frame #1 {
                                }
                                }
                                }
                                frame #2 {
                                n203 = for {
                                N: 9 -> [_]
                                tunnel: w707 -> [w726]
                                tunnel: w709 -> [w723]
                                tunnel: w714 -> [w724]
                                tunnel: w713 -> [w722]
                                tunnel: w706 -> [w725]
                                tunnel: [w724] -> w712
                                tunnel: [w723] -> w711
                                tunnel: [w722] -> w710
                                tunnel: w705 -> [w715]
                                i -> [w719]
                                n204 = property on="odd/even indicator" class="Bool (strict)"() -> ("Value"=w716:bool)  [unwired: 2 in, 2 out]
                                n205 = case shown="False" w716 {
                                tunnel: [i32[] [2, 2, 1, 1, 1, 0, 0, 0, 0, 2, 2, 2, 2, 2, 0] i32[] [0, 0, 1, 1, 1, 2, 2, 2, 2, 2, 2, 2, 2, 2, 0]] -> w721
                                tunnel: [i32[] [1, 0, 2, 1, 0, 2, 1, 0, 0, 0, 1, 2, 3, 4, 0] i32[] [1, 2, 0, 1, 2, 0, 1, 2, 2, 0, 1, 2, 3, 4, 0]] -> w720
                                frame False {
                                }
                                frame True {
                                }
                                }
                                n206 = flat-sequence {
                                tunnel: w726 -> [w735]
                                tunnel: w725 -> [w739]
                                tunnel: w724 -> [w738]
                                tunnel: w723 -> [w737]
                                tunnel: w722 -> [w736]
                                tunnel: w718 -> [w733]
                                tunnel: w717 -> [w732]
                                tunnel: w715 -> [w731]
                                frame #0 {
                                n207 = Index Array(array=w735, index (row)=w733, index (col)=w732) -> (element=w734:dbl)
                                n208 = call "take image.vi"("Voltage"=w734, "Exposure time"=w739, "expose any"=w731, "Busy out"=w736, "Exp In"=w737, "Galvo"=w738) -> ()  [unwired: 6 in]
                                }
                                frame #1 {
                                n209 = property on="Settle time" class="DigNum (strict)"() -> ("Value"=w740:u32)  [unwired: 2 in, 2 out]
                                n210 = Wait (ms)(milliseconds to wait=w740) -> ()  [unwired: 1 out]
                                }
                                }
                                n211 = Index Array(array=w720, index=w719) -> (element=w718:i32)
                                n212 = Index Array(array=w721, index=w719) -> (element=w717:i32)
                                }
                                }
                                frame #3 {
                                n213 = property on="acquire 488" class="Bool (strict)"() -> ("Value"=w744:bool)  [unwired: 2 in, 2 out]
                                n214 = property on="acquire 405" class="Bool (strict)"() -> ("Value"=w745:bool)  [unwired: 2 in, 2 out]
                                n215 = property on="acquire 640" class="Bool (strict)"() -> ("Value"=w743:bool)  [unwired: 2 in, 2 out]
                                n216 = Or(x=w744, y=w745) -> (x .or. y?=w742:bool)
                                n217 = Or(x=w742, y=w743) -> (x .or. y?=w741:bool)
                                n218 = case shown="False" w741 {
                                tunnel: w748 -> [_ w749]
                                frame False {
                                }
                                frame True {
                                n219 = call-poly <vilib>:"DAQmx Write.vi"("task/channels in"=w749, "data"=FALSE) -> ()  [unwired: 11 in, 3 out]
                                }
                                }
                                n220 = property on="odd/even indicator" class="Bool (strict)"() -> ("Value"=w747:bool)  [unwired: 2 in, 2 out]
                                n221 = Not(x=w747) -> (.not. x?=w746:bool)
                                n222 = property on="odd/even indicator" class="Bool (strict)"("Value"=w746) -> ()  [unwired: 2 in, 2 out]
                                }
                                }
                              }
                            }
                            n223 = case shown="True" "acquire 488" {
                              tunnel: w518 -> [w591 w597]
                              tunnel: w516 -> [w589 w601]
                              tunnel: w517 -> [w590 w602]
                              tunnel: [w591 w599] -> _
                              tunnel: [w590 w600] -> _
                              tunnel: [w589 w598] -> _
                              tunnel: w513 -> [_ _]
                              tunnel: w507 -> [_ w594]
                              tunnel: w510 -> [_ w593]
                              tunnel: w504 -> [_ w592]
                              frame False {
                              }
                              frame True {
                                n224 = property on="488 voltages" class="Arr (strict)"() -> ("Value"=w595:dbl[][])  [unwired: 2 in, 2 out]
                                n225 = stacked-sequence {
                                seq-local: [_ w611 _ _] -> [_ _ w632 _]
                                seq-local: [_ w610 _ _] -> [_ _ w631 _]
                                seq-local: [_ w609 _ _] -> [_ _ w627 _]
                                seq-local: [_ w608 _ _] -> [_ _ w625 _]
                                seq-local: [_ w607 _ _] -> [_ _ w624 _]
                                tunnel: w602 -> [_ w611 _ _]
                                tunnel: w601 -> [_ w610 _ _]
                                tunnel: w597 -> [_ w609 _ _]
                                tunnel: w595 -> [_ w608 _ _]
                                tunnel: "488 Exp" -> [_ w607 _ _]
                                tunnel: [_ _ w630 _] -> w600
                                tunnel: [_ _ w629 _] -> w599
                                tunnel: [_ _ w628 _] -> w598
                                tunnel: w595 -> [_ w606 _ _]
                                tunnel: w594 -> [_ w605 _ _]
                                tunnel: w593 -> [w603 _ _ w666]
                                tunnel: w592 -> [_ _ w623 _]
                                frame #0 {
                                n226 = call-poly <vilib>:"DAQmx Write.vi"("task/channels in"=w603, "data"=TRUE) -> ()  [unwired: 11 in, 3 out]
                                }
                                frame #1 {
                                n227 = flat-sequence {
                                tunnel: w606 -> [w618]
                                tunnel: w605 -> [w616]
                                tunnel: [w617] -> _
                                frame #0 {
                                n228 = property on="odd/even indicator" class="Bool (strict)"() -> ("Value"=w612:bool)  [unwired: 2 in, 2 out]
                                n229 = case shown="False" w612 {
                                tunnel: [2 0] -> w614
                                tunnel: [2 0] -> w613
                                frame False {
                                }
                                frame True {
                                }
                                }
                                n230 = Index Array(array=w618, index (row)=w614, index (col)=w613) -> (element=w615:dbl)
                                n231 = call-poly <vilib>:"DAQmx Write.vi"("task/channels in"=w616, "data"=w615) -> ("task out"=w617:refnum<k21>)  [unwired: 11 in, 2 out]
                                }
                                }
                                }
                                frame #2 {
                                n232 = for {
                                N: 9 -> [_]
                                tunnel: w625 -> [w644]
                                tunnel: w627 -> [w642]
                                tunnel: w632 -> [w643]
                                tunnel: w631 -> [w641]
                                tunnel: [w643] -> w630
                                tunnel: [w642] -> w629
                                tunnel: [w641] -> w628
                                tunnel: w624 -> [w640]
                                tunnel: w623 -> [w633]
                                i -> [w639]
                                n233 = property on="odd/even indicator" class="Bool (strict)"() -> ("Value"=w634:bool)  [unwired: 2 in, 2 out]
                                n234 = case shown="True" w634 {
                                tunnel: [i32[] [2, 2, 1, 1, 1, 0, 0, 0, 0, 2, 2, 2, 2, 2, 0] i32[] [0, 0, 1, 1, 1, 2, 2, 2, 2, 2, 2, 2, 2, 2, 0]] -> w635
                                tunnel: [i32[] [1, 0, 2, 1, 0, 2, 1, 0, 0, 0, 1, 2, 3, 4, 0] i32[] [1, 2, 0, 1, 2, 0, 1, 2, 2, 0, 1, 2, 3, 4, 0]] -> w636
                                frame False {
                                }
                                frame True {
                                }
                                }
                                n235 = Index Array(array=w636, index=w639) -> (element=w638:i32)
                                n236 = Index Array(array=w635, index=w639) -> (element=w637:i32)
                                n237 = flat-sequence {
                                tunnel: w644 -> [w653]
                                tunnel: w640 -> [w657]
                                tunnel: w643 -> [w656]
                                tunnel: w642 -> [w655]
                                tunnel: w641 -> [w654]
                                tunnel: w638 -> [w651]
                                tunnel: w637 -> [w650]
                                tunnel: w633 -> [w649]
                                frame #0 {
                                n238 = Index Array(array=w653, index (row)=w651, index (col)=w650) -> (element=w652:dbl)
                                n239 = call "take image.vi"("Voltage"=w652, "Exposure time"=w657, "expose any"=w649, "Busy out"=w654, "Exp In"=w655, "Galvo"=w656) -> ()  [unwired: 6 in]
                                }
                                frame #1 {
                                n240 = property on="Settle time" class="DigNum (strict)"() -> ("Value"=w658:u32)  [unwired: 2 in, 2 out]
                                n241 = Wait (ms)(milliseconds to wait=w658) -> ()  [unwired: 1 out]
                                }
                                }
                                }
                                }
                                frame #3 {
                                n242 = property on="acquire 561" class="Bool (strict)"() -> ("Value"=w662:bool)  [unwired: 2 in, 2 out]
                                n243 = property on="acquire 405" class="Bool (strict)"() -> ("Value"=w661:bool)  [unwired: 2 in, 2 out]
                                n244 = property on="acquire 640" class="Bool (strict)"() -> ("Value"=w663:bool)  [unwired: 2 in, 2 out]
                                n245 = property on="odd/even indicator" class="Bool (strict)"() -> ("Value"=w664:bool)  [unwired: 2 in, 2 out]
                                n246 = Not(x=w664) -> (.not. x?=w665:bool)
                                n247 = Or(x=w662, y=w661) -> (x .or. y?=w660:bool)
                                n248 = property on="odd/even indicator" class="Bool (strict)"("Value"=w665) -> ()  [unwired: 2 in, 2 out]
                                n249 = Or(x=w660, y=w663) -> (x .or. y?=w659:bool)
                                n250 = case shown="True" w659 {
                                tunnel: w666 -> [_ w667]
                                frame False {
                                }
                                frame True {
                                n251 = call-poly <vilib>:"DAQmx Write.vi"("task/channels in"=w667, "data"=FALSE) -> ()  [unwired: 11 in, 3 out]
                                }
                                }
                                }
                                }
                              }
                            }
                            n252 = case shown="True" "acquire 405" {
                              tunnel: w509 -> [_ w532]
                              tunnel: w507 -> [_ w530]
                              tunnel: w506 -> [_ w528]
                              tunnel: w505 -> [_ w527]
                              tunnel: w504 -> [_ w526]
                              frame False {
                              }
                              frame True {
                                n253 = property on="405 voltages" class="Arr (strict)"() -> ("Value"=w531:dbl[][])  [unwired: 2 in, 2 out]
                                n254 = stacked-sequence {
                                tunnel: w531 -> [_ w536 w551 _]
                                tunnel: w530 -> [_ w535 w550 _]
                                tunnel: [_ _ _ w586] -> _
                                tunnel: w532 -> [w533 _ _ w586]
                                tunnel: "405 Exp" -> [_ _ w549 _]
                                tunnel: w528 -> [_ _ w548 _]
                                tunnel: w527 -> [_ _ w547 _]
                                tunnel: w526 -> [_ _ w546 _]
                                frame #0 {
                                n255 = call-poly <vilib>:"DAQmx Write.vi"("task/channels in"=w533, "data"=TRUE) -> ()  [unwired: 11 in, 3 out]
                                }
                                frame #1 {
                                n256 = flat-sequence {
                                tunnel: w536 -> [w540]
                                tunnel: [w539] -> w537
                                tunnel: w535 -> [w538]
                                tunnel: [w545] -> _
                                tunnel: w537 -> [w545]
                                frame #0 {
                                n257 = Index Array(array=w540, index (row)=0, index (col)=0) -> (element=w541:dbl)
                                n258 = call-poly <vilib>:"DAQmx Write.vi"("task/channels in"=w538, "data"=w541) -> ("task out"=w539:refnum<k21>)  [unwired: 11 in, 2 out]
                                }
                                frame #1 {
                                n259 = Wait (ms)(milliseconds to wait=50) -> ()  [unwired: 1 out]
                                }
                                }
                                }
                                frame #2 {
                                n260 = for {
                                N: 9 -> [_]
                                tunnel: w551 -> [w562]
                                tunnel: w550 -> [w561]
                                tunnel: w549 -> [w560]
                                tunnel: w548 -> [w559]
                                tunnel: w547 -> [w558]
                                tunnel: w546 -> [w553]
                                i -> [w557]
                                n261 = property on="odd/even indicator" class="Bool (strict)"() -> ("Value"=w554:bool)  [unwired: 2 in, 2 out]
                                n262 = case shown="True" w554 {
                                tunnel: [i32[] [2, 2, 1, 1, 1, 0, 0, 0, 0, 2, 2, 2, 2, 2, 0] i32[] [0, 0, 1, 1, 1, 2, 2, 2, 2, 2, 2, 2, 2, 2, 0]] -> w556
                                tunnel: [i32[] [1, 0, 2, 1, 0, 2, 1, 0, 0, 0, 1, 2, 3, 4, 0] i32[] [1, 2, 0, 1, 2, 0, 1, 2, 2, 0, 1, 2, 3, 4, 0]] -> w555
                                frame False {
                                }
                                frame True {
                                }
                                }
                                n263 = flat-sequence {
                                tunnel: w564 -> [w576]
                                tunnel: w563 -> [w575]
                                tunnel: w562 -> [w574]
                                tunnel: w561 -> [w573]
                                tunnel: w560 -> [w572]
                                tunnel: w559 -> [w571]
                                tunnel: w558 -> [w570]
                                tunnel: w553 -> [w569]
                                frame #0 {
                                n264 = Index Array(array=w574, index (row)=w576, index (col)=w575) -> (element=w577:dbl)
                                n265 = call "take image.vi"("Voltage"=w577, "Exposure time"=w572, "expose any"=w569, "Busy out"=w570, "Exp In"=w571, "Galvo"=w573) -> ()  [unwired: 6 in]
                                }
                                frame #1 {
                                n266 = property on="Settle time" class="DigNum (strict)"() -> ("Value"=w578:u32)  [unwired: 2 in, 2 out]
                                n267 = Wait (ms)(milliseconds to wait=w578) -> ()  [unwired: 1 out]
                                }
                                }
                                n268 = Index Array(array=w555, index=w557) -> (element=w564:i32)
                                n269 = Index Array(array=w556, index=w557) -> (element=w563:i32)
                                }
                                }
                                frame #3 {
                                n270 = property on="acquire 561" class="Bool (strict)"() -> ("Value"=w581:bool)  [unwired: 2 in, 2 out]
                                n271 = property on="acquire 488" class="Bool (strict)"() -> ("Value"=w582:bool)  [unwired: 2 in, 2 out]
                                n272 = property on="acquire 640" class="Bool (strict)"() -> ("Value"=w580:bool)  [unwired: 2 in, 2 out]
                                n273 = Or(x=w581, y=w582) -> (x .or. y?=w583:bool)
                                n274 = property on="odd/even indicator" class="Bool (strict)"() -> ("Value"=w585:bool)  [unwired: 2 in, 2 out]
                                n275 = Or(x=w583, y=w580) -> (x .or. y?=w579:bool)
                                n276 = Not(x=w585) -> (.not. x?=w584:bool)
                                n277 = property on="odd/even indicator" class="Bool (strict)"("Value"=w584) -> ()  [unwired: 2 in, 2 out]
                                n278 = case shown="True" w579 {
                                tunnel: w586 -> [_ w587]
                                frame False {
                                }
                                frame True {
                                n279 = call-poly <vilib>:"DAQmx Write.vi"("task/channels in"=w587, "data"=FALSE) -> ()  [unwired: 11 in, 3 out]
                                }
                                }
                                }
                                }
                              }
                            }
                          }
                          frame "fast sequence" {
                            # "561"
                            # "488"
                            # "fast sequence"
                            n280 = property on="647 Exp" class="DigNum (strict)"() -> ("Value"=w837:dbl)  [unwired: 2 in, 2 out]
                            n281 = property on="647 voltages" class="Arr (strict)"() -> ("Value"=w840:dbl[][])  [unwired: 2 in, 2 out]
                            n282 = stacked-sequence {
                              seq-local: [_ w922 _ _] -> [_ _ w940 _]
                              seq-local: [_ w921 _ _] -> [_ _ w939 _]
                              seq-local: [_ w920 _ _] -> [_ _ w938 _]
                              seq-local: [_ w919 _ _] -> [_ _ w934 _]
                              seq-local: [_ w918 _ _] -> [_ _ w933 _]
                              tunnel: w848 -> [_ w922 _ _]
                              tunnel: w843 -> [_ w921 _ _]
                              tunnel: w847 -> [_ w920 _ _]
                              tunnel: w840 -> [_ w919 _ _]
                              tunnel: w837 -> [_ w918 _ _]
                              tunnel: [_ _ w937 _] -> w845
                              tunnel: [_ _ w936 _] -> w844
                              tunnel: [_ _ w935 _] -> w846
                              tunnel: w840 -> [_ w916 _ _]
                              tunnel: w843 -> [_ w915 _ _]
                              tunnel: w842 -> [w913 _ _ w971]
                              tunnel: w836 -> [w911 _ _ w969]
                              tunnel: w834 -> [_ _ w931 _]
                              frame #0 {
                                n283 = VISA Write(VISA resource name=w913, write buffer="la on\r" ("format string")) -> ()  [unwired: 1 in, 3 out]
                                n284 = call-poly <vilib>:"DAQmx Write.vi"("task/channels in"=w911, "data"=TRUE) -> ()  [unwired: 11 in, 3 out]
                              }
                              frame #1 {
                                n285 = flat-sequence {
                                tunnel: [w923] -> _
                                tunnel: w916 -> [w925]
                                tunnel: [w924] -> w917
                                tunnel: w915 -> [w923]
                                tunnel: [w930] -> _
                                tunnel: w917 -> [w930]
                                frame #0 {
                                n286 = Index Array(array=w925, index (row)=0, index (col)=0) -> (element=w926:dbl)
                                n287 = call-poly <vilib>:"DAQmx Write.vi"("task/channels in"=w923, "data"=w926) -> ("task out"=w924:refnum<k21>)  [unwired: 11 in, 2 out]
                                }
                                frame #1 {
                                n288 = Wait (ms)(milliseconds to wait=50) -> ()  [unwired: 1 out]
                                }
                                }
                              }
                              frame #2 {
                                n289 = for {
                                N: 9 -> [_]
                                tunnel: w934 -> [w952]
                                tunnel: w940 -> [w949]
                                tunnel: w939 -> [w950]
                                tunnel: w938 -> [w948]
                                tunnel: w933 -> [w951]
                                tunnel: [w950] -> w937
                                tunnel: [w949] -> w936
                                tunnel: [w948] -> w935
                                tunnel: w931 -> [w941]
                                i -> [w946]
                                n290 = property on="odd/even indicator" class="Bool (strict)"() -> ("Value"=w944:bool)  [unwired: 2 in, 2 out]
                                n291 = case shown="False" w944 {
                                tunnel: [i32[] [2, 2, 1, 1, 1, 0, 0, 0, 0, 2, 2, 2, 2, 2, 0] i32[] [0, 0, 1, 1, 1, 2, 2, 2, 2, 2, 2, 2, 2, 2, 0]] -> w942
                                tunnel: [i32[] [1, 0, 2, 1, 0, 2, 1, 0, 0, 0, 1, 2, 3, 4, 0] i32[] [1, 2, 0, 1, 2, 0, 1, 2, 2, 0, 1, 2, 3, 4, 0]] -> w943
                                frame False {
                                }
                                frame True {
                                }
                                }
                                n292 = Index Array(array=w943, index=w946) -> (element=w947:i32)
                                n293 = flat-sequence {
                                tunnel: w952 -> [w961]
                                tunnel: w951 -> [w965]
                                tunnel: w950 -> [w964]
                                tunnel: w949 -> [w963]
                                tunnel: w948 -> [w962]
                                tunnel: w945 -> [w959]
                                tunnel: w947 -> [w958]
                                tunnel: w941 -> [w957]
                                frame #0 {
                                n294 = Index Array(array=w961, index (row)=w958, index (col)=w959) -> (element=w960:dbl)
                                n295 = call "take image.vi"("Voltage"=w960, "Exposure time"=w965, "expose any"=w957, "Busy out"=w962, "Exp In"=w963, "Galvo"=w964) -> ()  [unwired: 6 in]
                                }
                                frame #1 {
                                n296 = property on="Settle time" class="DigNum (strict)"() -> ("Value"=w966:u32)  [unwired: 2 in, 2 out]
                                n297 = Wait (ms)(milliseconds to wait=w966) -> ()  [unwired: 1 out]
                                }
                                }
                                n298 = Index Array(array=w942, index=w946) -> (element=w945:i32)
                                }
                              }
                              frame #3 {
                                n299 = property on="odd/even indicator" class="Bool (strict)"() -> ("Value"=w967:bool)  [unwired: 2 in, 2 out]
                                n300 = Not(x=w967) -> (.not. x?=w968:bool)
                                n301 = property on="odd/even indicator" class="Bool (strict)"("Value"=w968) -> ()  [unwired: 2 in, 2 out]
                                n302 = VISA Write(VISA resource name=w971, write buffer="la off\r" ("format string")) -> ()  [unwired: 1 in, 3 out]
                                n303 = call-poly <vilib>:"DAQmx Write.vi"("task/channels in"=w969, "data"=FALSE) -> ()  [unwired: 11 in, 3 out]
                              }
                            }
                            n304 = property on="561 voltages" class="Arr (strict)"() -> ("Value"=w839:dbl[][])  [unwired: 2 in, 2 out]
                            n305 = property on="561 Exp" class="DigNum (strict)"() -> ("Value"=w838:dbl)  [unwired: 2 in, 2 out]
                            n306 = stacked-sequence {
                              seq-local: [_ w860 _ _] -> [_ _ w878 _]
                              seq-local: [_ w859 _ _] -> [_ _ w877 _]
                              seq-local: [_ w858 _ _] -> [_ _ w873 _]
                              seq-local: [_ w857 _ _] -> [_ _ w871 _]
                              seq-local: [_ w856 _ _] -> [_ _ w870 _]
                              tunnel: w845 -> [_ w860 _ _]
                              tunnel: w846 -> [_ w859 _ _]
                              tunnel: w844 -> [_ w858 _ _]
                              tunnel: w839 -> [_ w857 _ _]
                              tunnel: w838 -> [_ w856 _ _]
                              tunnel: [_ _ w876 _] -> _
                              tunnel: [_ _ w875 _] -> _
                              tunnel: [_ _ w874 _] -> _
                              tunnel: w839 -> [_ w854 _ _]
                              tunnel: w843 -> [_ w853 _ _]
                              tunnel: w841 -> [w852 _ _ w909]
                              tunnel: w835 -> [w849 _ _ w907]
                              tunnel: w834 -> [_ _ w869 _]
                              frame #0 {
                                n307 = call-poly <vilib>:"DAQmx Write.vi"("task/channels in"=w852, "data"=TRUE) -> ()  [unwired: 11 in, 3 out]
                                n308 = call-poly <vilib>:"DAQmx Write.vi"("task/channels in"=w849, "data"=TRUE) -> ()  [unwired: 11 in, 3 out]
                              }
                              frame #1 {
                                n309 = flat-sequence {
                                tunnel: w854 -> [w863]
                                tunnel: [w862] -> w855
                                tunnel: w853 -> [w861]
                                tunnel: [w868] -> _
                                tunnel: w855 -> [w868]
                                frame #0 {
                                n310 = Index Array(array=w863, index (row)=0, index (col)=0) -> (element=w864:dbl)
                                n311 = call-poly <vilib>:"DAQmx Write.vi"("task/channels in"=w861, "data"=w864) -> ("task out"=w862:refnum<k21>)  [unwired: 11 in, 2 out]
                                }
                                frame #1 {
                                n312 = Wait (ms)(milliseconds to wait=50) -> ()  [unwired: 1 out]
                                }
                                }
                              }
                              frame #2 {
                                n313 = for {
                                N: 9 -> [_]
                                tunnel: w871 -> [w890]
                                tunnel: w873 -> [w887]
                                tunnel: w878 -> [w888]
                                tunnel: w877 -> [w886]
                                tunnel: w870 -> [w889]
                                tunnel: [w888] -> w876
                                tunnel: [w887] -> w875
                                tunnel: [w886] -> w874
                                tunnel: w869 -> [w879]
                                i -> [w885]
                                n314 = property on="odd/even indicator" class="Bool (strict)"() -> ("Value"=w880:bool)  [unwired: 2 in, 2 out]
                                n315 = case shown="True" w880 {
                                tunnel: [i32[] [2, 2, 1, 1, 1, 0, 0, 0, 0, 2, 2, 2, 2, 2, 0] i32[] [0, 0, 1, 1, 1, 2, 2, 2, 2, 2, 2, 2, 2, 2, 0]] -> w881
                                tunnel: [i32[] [1, 0, 2, 1, 0, 2, 1, 0, 0, 0, 1, 2, 3, 4, 0] i32[] [1, 2, 0, 1, 2, 0, 1, 2, 2, 0, 1, 2, 3, 4, 0]] -> w882
                                frame False {
                                }
                                frame True {
                                }
                                }
                                n316 = Index Array(array=w882, index=w885) -> (element=w884:i32)
                                n317 = Index Array(array=w881, index=w885) -> (element=w883:i32)
                                n318 = flat-sequence {
                                tunnel: w890 -> [w899]
                                tunnel: w889 -> [w903]
                                tunnel: w888 -> [w902]
                                tunnel: w887 -> [w901]
                                tunnel: w886 -> [w900]
                                tunnel: w884 -> [w897]
                                tunnel: w883 -> [w896]
                                tunnel: w879 -> [w895]
                                frame #0 {
                                n319 = Index Array(array=w899, index (row)=w897, index (col)=w896) -> (element=w898:dbl)
                                n320 = call "take image.vi"("Voltage"=w898, "Exposure time"=w903, "expose any"=w895, "Busy out"=w900, "Exp In"=w901, "Galvo"=w902) -> ()  [unwired: 6 in]
                                }
                                frame #1 {
                                n321 = property on="Settle time" class="DigNum (strict)"() -> ("Value"=w904:u32)  [unwired: 2 in, 2 out]
                                n322 = Wait (ms)(milliseconds to wait=w904) -> ()  [unwired: 1 out]
                                }
                                }
                                }
                              }
                              frame #3 {
                                n323 = call-poly <vilib>:"DAQmx Write.vi"("task/channels in"=w909, "data"=FALSE) -> ()  [unwired: 11 in, 3 out]
                                n324 = property on="odd/even indicator" class="Bool (strict)"() -> ("Value"=w906:bool)  [unwired: 2 in, 2 out]
                                n325 = call-poly <vilib>:"DAQmx Write.vi"("task/channels in"=w907, "data"=FALSE) -> ()  [unwired: 11 in, 3 out]
                                n326 = Not(x=w906) -> (.not. x?=w905:bool)
                                n327 = property on="odd/even indicator" class="Bool (strict)"("Value"=w905) -> ()  [unwired: 2 in, 2 out]
                              }
                            }
                          }
                          frame "optosplit" {
                            n328 = case shown="False" w974 {
                              tunnel: w977 -> [w983 w1020]
                              tunnel: w976 -> [w982 w1019]
                              tunnel: w975 -> [w981 w1018]
                              tunnel: w973 -> [_ w1012]
                              frame True {
                                w978 = 15
                                # "With optosplit"
                                n329 = flat-sequence {
                                tunnel: w981 -> [w987]
                                tunnel: w980 -> [w986]
                                tunnel: [w985] -> w984
                                tunnel: [w994] -> w979
                                tunnel: w984 -> [w994]
                                frame #0 {
                                n330 = Index Array(array=w986, index (row)=0, index (col)=0) -> (element=w988:dbl)
                                n331 = call-poly <vilib>:"DAQmx Write.vi"("task/channels in"=w987, "data"=w988) -> ("task out"=w985:refnum<k21>)  [unwired: 11 in, 2 out]
                                }
                                frame #1 {
                                n332 = property on="Settle time" class="DigNum (strict)"() -> ("Value"=w993:u32)  [unwired: 2 in, 2 out]
                                n333 = Add(x=w993, y=20) -> (x+y=w992:u32)
                                n334 = Wait (ms)(milliseconds to wait=w992) -> ()  [unwired: 1 out]
                                }
                                }
                                n335 = property on="561 voltages" class="Arr (strict)"() -> ("Value"=w980:dbl[][])  [unwired: 2 in, 2 out]
                                n336 = for {
                                N: w978 -> [_]
                                tunnel: w980 -> [w1002]
                                tunnel: w983 -> [w1005]
                                tunnel: w982 -> [w1004]
                                tunnel: w979 -> [w1003]
                                tunnel: w978 -> [_]
                                i -> [w998]
                                n337 = property on="Exposure time" class="DigNum (strict)"() -> ("Value"=w1001:dbl)  [unwired: 2 in, 2 out]
                                n338 = Index Array(array=i32[] [1, 2, 3, 4, 0, 1, 2, 3, 4, 0, 1, 2, 3, 4, 0], index=w998) -> (element=w996:i32)
                                n339 = Index Array(array=i32[] [0, 0, 0, 0, 1, 1, 1, 1, 1, 2, 2, 2, 2, 2, 0], index=w998) -> (element=w997:i32)
                                n340 = Index Array(array=w1002, index (row)=w996, index (col)=w997) -> (element=w995:dbl)
                                n341 = property on="Current voltage" class="DigNum (strict)"("Value"=w995) -> ()  [unwired: 2 in, 2 out]
                                n342 = flat-sequence {
                                tunnel: w1005 -> [w1010]
                                tunnel: w1004 -> [w1009]
                                tunnel: w995 -> [w1008]
                                tunnel: w1003 -> [w1007]
                                tunnel: w1001 -> [w1006]
                                frame #0 {
                                n343 = call "take image.vi"("Voltage"=w1008, "Exposure time"=w1006, "Busy out"=w1009, "Exp In"=w1010, "Galvo"=w1007) -> ()  [unwired: 7 in]
                                }
                                frame #1 {
                                n344 = property on="Settle time" class="DigNum (strict)"() -> ("Value"=w1011:u32)  [unwired: 2 in, 2 out]
                                n345 = Wait (ms)(milliseconds to wait=w1011) -> ()  [unwired: 1 out]
                                }
                                }
                                }
                              }
                              frame False {
                                w1015 = 9
                                # "With optosplit"
                                n346 = flat-sequence {
                                tunnel: w1018 -> [w1027]
                                tunnel: w1017 -> [w1026]
                                tunnel: [w1025] -> w1021
                                tunnel: [w1036] -> w1016
                                tunnel: w1021 -> [w1036]
                                frame #0 {
                                n347 = property on="odd/even indicator" class="Bool (strict)"() -> ("Value"=w1024:bool)  [unwired: 2 in, 2 out]
                                n348 = case shown="False" w1024 {
                                tunnel: [2 0] -> w1023
                                tunnel: [2 0] -> w1022
                                frame False {
                                }
                                frame True {
                                }
                                }
                                n349 = Index Array(array=w1026, index (row)=w1023, index (col)=w1022) -> (element=w1028:dbl)
                                n350 = call-poly <vilib>:"DAQmx Write.vi"("task/channels in"=w1027, "data"=w1028) -> ("task out"=w1025:refnum<k21>)  [unwired: 11 in, 2 out]
                                }
                                frame #1 {
                                n351 = property on="Settle time" class="DigNum (strict)"() -> ("Value"=w1035:u32)  [unwired: 2 in, 2 out]
                                n352 = Add(x=w1035, y=20) -> (x+y=w1034:u32)
                                n353 = Wait (ms)(milliseconds to wait=w1034) -> ()  [unwired: 1 out]
                                }
                                }
                                n354 = property on="561 voltages" class="Arr (strict)"() -> ("Value"=w1017:dbl[][])  [unwired: 2 in, 2 out]
                                n355 = for {
                                N: w1015 -> [_]
                                tunnel: w1017 -> [w1046]
                                tunnel: w1020 -> [w1049]
                                tunnel: w1019 -> [w1048]
                                tunnel: w1016 -> [w1047]
                                tunnel: w1015 -> [_]
                                tunnel: [w1038] -> w1013
                                tunnel: w1012 -> [w1037]
                                i -> [w1044]
                                n356 = property on="odd/even indicator" class="Bool (strict)"() -> ("Value"=w1038:bool)  [unwired: 2 in, 2 out]
                                n357 = property on="Exposure time" class="DigNum (strict)"() -> ("Value"=w1045:dbl)  [unwired: 2 in, 2 out]
                                n358 = case shown="False" w1038 {
                                tunnel: [i32[] [2, 2, 1, 1, 1, 0, 0, 0, 0, 2, 2, 2, 2, 2, 0] i32[] [0, 0, 1, 1, 1, 2, 2, 2, 2, 2, 2, 2, 2, 2, 0]] -> w1039
                                tunnel: [i32[] [1, 0, 2, 1, 0, 2, 1, 0, 0, 0, 1, 2, 3, 4, 0] i32[] [1, 2, 0, 1, 2, 0, 1, 2, 2, 0, 1, 2, 3, 4, 0]] -> w1040
                                frame False {
                                }
                                frame True {
                                }
                                }
                                n359 = Index Array(array=w1040, index=w1044) -> (element=w1042:i32)
                                n360 = Index Array(array=w1039, index=w1044) -> (element=w1043:i32)
                                n361 = Index Array(array=w1046, index (row)=w1042, index (col)=w1043) -> (element=w1041:dbl)
                                n362 = property on="Current voltage" class="DigNum (strict)"("Value"=w1041) -> ()  [unwired: 2 in, 2 out]
                                n363 = flat-sequence {
                                tunnel: w1049 -> [w1059]
                                tunnel: w1048 -> [w1058]
                                tunnel: w1041 -> [w1057]
                                tunnel: w1047 -> [w1056]
                                tunnel: w1045 -> [w1055]
                                tunnel: w1037 -> [w1054]
                                frame #0 {
                                n364 = call "take image.vi"("Voltage"=w1057, "Exposure time"=w1055, "expose any"=w1054, "Busy out"=w1058, "Exp In"=w1059, "Galvo"=w1056) -> ()  [unwired: 6 in]
                                }
                                frame #1 {
                                n365 = property on="Settle time" class="DigNum (strict)"() -> ("Value"=w1060:u32)  [unwired: 2 in, 2 out]
                                n366 = Wait (ms)(milliseconds to wait=w1060) -> ()  [unwired: 1 out]
                                }
                                }
                                }
                                n367 = Not(x=w1013) -> (.not. x?=w1014:bool)
                                n368 = property on="odd/even indicator" class="Bool (strict)"("Value"=w1014) -> ()  [unwired: 2 in, 2 out]
                              }
                            }
                          }
                          frame "rolling SIM" {
                            w1064 = 0 ("index")
                            # "Rolling SIM"
                            n369 = Build Array("short delay", "short delay", "long delay") -> (w1065:dbl[])
                            n370 = Insert Into Array(array=w1065, index=w1064, new element=w1065) -> (w1066:dbl[])
                            n371 = Insert Into Array(array=w1066, index=w1064, new element=w1066) -> (w1061:dbl[])
                            n372 = property on="561 voltages" class="Arr (strict)"() -> ("Value"=w1072:dbl[][])  [unwired: 2 in, 2 out]
                            n373 = for {
                              N: 12 -> [_]
                              tunnel: w1072 -> [w1077]
                              tunnel: w1074 -> [w1088]
                              tunnel: w1073 -> [w1087]
                              tunnel: [w1080] -> w1069
                              tunnel: w1068 -> [w1079]
                              tunnel: w1067 -> [w1078]
                              tunnel: w1061 -> [w1075] mode=indexing
                              i -> [w1076]
                              n374 = property on="Exposure time" class="DigNum (strict)"() -> ("Value"=w1086:dbl)  [unwired: 2 in, 2 out]
                              n375 = Index Array(array=i32[] [1, 2, 0, 1, 2, 0, 1, 2, 0, 1, 2, 0, 3, 4, 0], index=w1076) -> (element=w1084:i32)
                              n376 = Index Array(array=i32[] [0, 0, 1, 1, 1, 2, 2, 2, 1, 1, 1, 0, 2, 2, 0], index=w1076) -> (element=w1085:i32)
                              n377 = Index Array(array=w1077, index (row)=w1084, index (col)=w1085) -> (element=w1083:dbl)
                              n378 = property on="Current voltage" class="DigNum (strict)"("Value"=w1083) -> ()  [unwired: 2 in, 2 out]
                              n379 = flat-sequence {
                                tunnel: w1088 -> [w1094]
                                tunnel: w1087 -> [w1090]
                                tunnel: w1083 -> [w1093]
                                tunnel: w1086 -> [w1092]
                                tunnel: w1079 -> [w1091]
                                tunnel: w1078 -> [w1089]
                                tunnel: w1075 -> [w1095]
                                frame #0 {
                                n380 = call "take image.vi"("Voltage"=w1093, "Exposure time"=w1092, "expose any"=w1091, "Busy out"=w1090, "Exp In"=w1094, "Galvo"=w1089) -> ()  [unwired: 6 in]
                                }
                                frame #1 {
                                n381 = Wait (ms)(milliseconds to wait=w1095) -> ()  [unwired: 1 out]
                                }
                              }
                              n382 = property on="odd/even indicator" class="Bool (strict)"() -> ("Value"=w1080:bool)  [unwired: 2 in, 2 out]
                            }
                            n383 = Not(x=w1069) -> (.not. x?=w1070:bool)
                            n384 = property on="odd/even indicator" class="Bool (strict)"("Value"=w1070) -> ()  [unwired: 2 in, 2 out]
                          }
                        }
                      }
                      frame #1 {
                        n385 = Greater?(x=w1099, y=1) -> (0:w1098:bool)
                        n386 = Greater?(x="Steps /um", y=0) -> (0:w1097:bool)
                        n387 = And(x=w1098, y=w1097) -> (x .and. y?=w1096:bool)
                        n388 = case shown="True" w1096 {
                          tunnel: w1104 -> [w1105 w1108]
                          tunnel: [w1105 w1107] -> w1103
                          tunnel: "Steps /um" -> [_ w1106]
                          frame False {
                          }
                          frame True {
                            n389 = flat-sequence {
                              tunnel: w1108 -> [w1116]
                              tunnel: [w1115] -> w1109
                              tunnel: w1106 -> [w1112]
                              tunnel: [w1119] -> w1107
                              tunnel: w1109 -> [w1119]
                              frame #0 {
                                n390 = Multiply(x=w1112, y=10.0) -> (x*y=w1110:dbl)
                                n391 = Format Into String "Format Into String"(format string="movrel\\sz=%f\\s\\r\\n", w1110) -> (resulting string=w1113:string)  [unwired: 2 in, 1 out]
                                "resulting string" <- w1113
                                n392 = VISA Write(VISA resource name=w1116, write buffer=w1113) -> (VISA resource name out=w1115:refnum<visa-resource-name>, error out=→"optosplit stage error":errorcluster)  [unwired: 1 in, 1 out]
                              }
                              frame #1 {
                                n393 = Wait (ms)(milliseconds to wait=20) -> ()  [unwired: 1 out]
                              }
                            }
                          }
                        }
                      }
                    }
                  }
                }
                frame #1 {
                  n394 = flat-sequence {
                    tunnel: w1135 -> [w1145]
                    tunnel: w1134 -> [w1144]
                    tunnel: w1133 -> [w1143]
                    tunnel: w1132 -> [w1142]
                    tunnel: [w1141] -> w1129
                    tunnel: [w1140] -> w1126
                    tunnel: [w1139] -> w1123
                    tunnel: [w1138] -> w1122
                    tunnel: w1136 -> [w1169]
                    tunnel: [w1168] -> w1130
                    tunnel: w1129 -> [w1168]
                    tunnel: [w1167] -> w1127
                    tunnel: w1126 -> [w1167]
                    tunnel: [w1166] -> w1124
                    tunnel: w1123 -> [w1166]
                    tunnel: w1122 -> [w1165]
                    tunnel: [w1165] -> w1120
                    tunnel: [w1183] -> w1131
                    tunnel: w1130 -> [w1183]
                    tunnel: [w1182] -> w1128
                    tunnel: w1127 -> [w1182]
                    tunnel: [w1181] -> w1125
                    tunnel: w1124 -> [w1181]
                    tunnel: [w1180] -> w1121
                    tunnel: w1120 -> [w1180]
                    tunnel: w1131 -> [w1190]
                    tunnel: w1128 -> [w1189]
                    tunnel: w1125 -> [w1188]
                    tunnel: w1121 -> [w1187]
                    frame #0 {
                      n395 = case shown="False" FALSE {
                        tunnel: w1145 -> [w1149 w1157]
                        tunnel: w1144 -> [w1148 w1156]
                        tunnel: w1143 -> [w1147 w1155]
                        tunnel: w1142 -> [w1146 w1154]
                        tunnel: [w1146 w1153] -> w1141
                        tunnel: [w1147 w1152] -> w1140
                        tunnel: [w1148 w1151] -> w1139
                        tunnel: [w1149 w1150] -> w1138
                        frame False {
                        }
                        frame True {
                          n396 = call-poly <vilib>:"DAQmx Write.vi"("task/channels in"=w1156, "data"=FALSE) -> ("task out"=w1151:refnum<k21>)  [unwired: 11 in, 2 out]
                          n397 = call-poly <vilib>:"DAQmx Write.vi"("task/channels in"=w1157, "data"=FALSE) -> ("task out"=w1150:refnum<k21>)  [unwired: 11 in, 2 out]
                          n398 = call-poly <vilib>:"DAQmx Write.vi"("task/channels in"=w1155, "data"=FALSE) -> ("task out"=w1152:refnum<k21>)  [unwired: 11 in, 2 out]
                          n399 = VISA Write(VISA resource name=w1154, write buffer="la off\r" ("format string")) -> (VISA resource name out=w1153:refnum<visa-resource-name>)  [unwired: 1 in, 2 out]
                        }
                      }
                    }
                    frame #1 {
                      n400 = property on="z-slices" class="DigNum (strict)"() -> ("Value"=w1163:dbl)  [unwired: 2 in, 2 out]
                      n401 = property on="Optosplit" class="RadioBtnsControl (strict)" props=["Value"]() -> ()  [unwired: 2 in, 3 out]
                      n402 = Greater?(x=w1163, y=1) -> (0:w1162:bool)
                      n403 = case shown="False" w1162 {
                        tunnel: w1169 -> [_ w1176]
                        frame False {
                        }
                        frame True {
                          n404 = property on="z-slices" class="DigNum (strict)"() -> ("Value"=w1174:dbl)  [unwired: 2 in, 2 out]
                          n405 = property on="Steps /um" class="DigNum (strict)"() -> ("Value"=w1175:dbl)  [unwired: 2 in, 2 out]
                          n406 = Negate(x=w1175) -> (-x=w1173:dbl)
                          n407 = Multiply(x=w1173, y=w1174) -> (x*y=w1172:dbl)
                          n408 = Multiply(x=w1172, y=10.0) -> (x*y=w1170:dbl)
                          n409 = Format Into String "Format Into String"(format string="movrel\\sz=%f\\s\\r\\n", w1170) -> (resulting string=w1178:string)  [unwired: 2 in, 1 out]
                          "resulting string 2" <- w1178
                          n410 = VISA Write(VISA resource name=w1176, write buffer=w1178) -> (error out=→"stage error":errorcluster)  [unwired: 1 in, 2 out]
                        }
                      }
                    }
                    frame #2 {
                      n411 = Multiply(x="interval /s", y=1000.0) -> (x*y=w1186:dbl)
                      n412 = Wait (ms)(milliseconds to wait=w1186) -> ()  [unwired: 1 out]
                    }
                    frame #3 {
                      n413 = property on="Optosplit" class="RadioBtnsControl (strict)"() -> ("Value"=w1191:T2)  [unwired: 2 in, 2 out]
                      n414 = disable-structure shown="Disabled" {
                        disable-tunnel: w1191 -> [w1196 _]
                        disable-tunnel: w1190 -> [w1195 _]
                        disable-tunnel: w1189 -> [w1194 _]
                        disable-tunnel: w1188 -> [w1193 _]
                        disable-tunnel: w1187 -> [w1192 _]
                        frame Disabled {
                          n415 = case shown="\"rolling SIM\"" w1196 {
                            tunnel: w1195 -> [_ w1200 w1208 w1216]
                            tunnel: w1194 -> [_ w1199 w1207 w1215]
                            tunnel: w1193 -> [_ w1198 w1206 w1214]
                            tunnel: w1192 -> [_ w1197 w1205 w1213]
                            frame "sequential", Default {
                            }
                            frame "optosplit" {
                              n416 = call-poly <vilib>:"DAQmx Write.vi"("task/channels in"=w1198, "data"=TRUE) -> ()  [unwired: 11 in, 3 out]
                              n417 = call-poly <vilib>:"DAQmx Write.vi"("task/channels in"=w1197, "data"=TRUE) -> ()  [unwired: 11 in, 3 out]
                              n418 = call-poly <vilib>:"DAQmx Write.vi"("task/channels in"=w1199, "data"=TRUE) -> ()  [unwired: 11 in, 3 out]
                              n419 = VISA Write(VISA resource name=w1200, write buffer="la on\r" ("format string")) -> ()  [unwired: 1 in, 3 out]
                            }
                            frame "rolling SIM" {
                              n420 = call-poly <vilib>:"DAQmx Write.vi"("task/channels in"=w1206, "data"=TRUE) -> ()  [unwired: 11 in, 3 out]
                              n421 = call-poly <vilib>:"DAQmx Write.vi"("task/channels in"=w1205, "data"=TRUE) -> ()  [unwired: 11 in, 3 out]
                              n422 = call-poly <vilib>:"DAQmx Write.vi"("task/channels in"=w1207, "data"=TRUE) -> ()  [unwired: 11 in, 3 out]
                              n423 = VISA Write(VISA resource name=w1208, write buffer="la on\r" ("format string")) -> ()  [unwired: 1 in, 3 out]
                            }
                            frame "fast sequence" {
                              n424 = call-poly <vilib>:"DAQmx Write.vi"("task/channels in"=w1214, "data"=TRUE) -> ()  [unwired: 11 in, 3 out]
                              n425 = call-poly <vilib>:"DAQmx Write.vi"("task/channels in"=w1213, "data"=TRUE) -> ()  [unwired: 11 in, 3 out]
                              n426 = call-poly <vilib>:"DAQmx Write.vi"("task/channels in"=w1215, "data"=TRUE) -> ()  [unwired: 11 in, 3 out]
                              n427 = VISA Write(VISA resource name=w1216, write buffer="la on\r" ("format string")) -> ()  [unwired: 1 in, 3 out]
                            }
                          }
                        }
                        frame Enabled {
                        }
                      }
                    }
                  }
                }
              }
              n428 = property on="Go SIM" class="Bool (strict)"() -> ("Value"=w436:bool)  [unwired: 2 in, 2 out]
              n429 = Not(x=w436) -> (.not. x?=w435:bool)
            }
          }
          frame #3 {
            w1225 = FALSE
            n430 = property on="Go SIM" class="Bool (strict)"("Value"=FALSE ("Go SIM")) -> ()  [unwired: 2 in, 2 out]
            n431 = property on="Tab Control" class="TabCtl (strict)"("DisabledEnum"=T4."Enabled" ("Disabled")) -> ()  [unwired: 2 in, 2 out]
            n432 = VISA Write(VISA resource name=w1222, write buffer="L 0\n" ("format string")) -> ()  [unwired: 1 in, 3 out]
            n433 = call-poly <vilib>:"DAQmx Write.vi"("task/channels in"=w1228, "data"=FALSE) -> ()  [unwired: 11 in, 3 out]
            n434 = call-poly <vilib>:"DAQmx Write.vi"("task/channels in"=w1229, "data"=FALSE) -> ()  [unwired: 11 in, 3 out]
            n435 = VISA Write(VISA resource name=w1226, write buffer="la off\r" ("format string")) -> ()  [unwired: 1 in, 3 out]
            n436 = property on="561" class="Bool (strict)"("Value"=w1225) -> ()  [unwired: 2 in, 2 out]
            n437 = property on="488" class="Bool (strict)"("Value"=w1225) -> ()  [unwired: 2 in, 2 out]
            n438 = property on="405" class="Bool (strict)"("Value"=w1225) -> ()  [unwired: 2 in, 2 out]
            n439 = property on="647" class="Bool (strict)"("Value"=w1225) -> ()  [unwired: 2 in, 2 out]
          }
        }
      }
    }
    n440 = property on="stop" class="Bool (strict)"() -> ("Value"=w255:bool)  [unwired: 2 in, 2 out]
    n441 = Wait (ms)(milliseconds to wait=u32 100) -> ()  [unwired: 1 out]
  }
  n442 = VISA Write(VISA resource name=w17, write buffer=w23) -> (VISA resource name out=w16:refnum<visa-resource-name>)  [unwired: 1 in, 2 out]
  n443 = VISA Write(VISA resource name=w56, write buffer="en 1\r" ("format string")) -> (VISA resource name out=w55:refnum<visa-resource-name>)  [unwired: 1 in, 2 out]
  n444 = while {
    tunnel: w91 -> [w1242]
    tunnel: w92 -> [w1243]
    tunnel: [w1243] -> w81
    tunnel: [w1242] -> w80
    tunnel: w55 -> [w1238]
    tunnel: w54 -> [_]
    tunnel: [w1240] -> w61
    tunnel: [w1239] -> w60
    tunnel: w29 -> [w1236]
    tunnel: [w1236] -> w10
    tunnel: w25 -> [w1234]
    tunnel: w16 -> [w1233]
    tunnel: [w1233] -> w13
    stop <- w1241 stop-if-true
    w1235 = 100
    n445 = Wait (ms)(milliseconds to wait=u32 250) -> ()  [unwired: 1 out]
    n446 = event shown="[1] \"Jog Z\": Value Change" {
      selector: _ -> [_ _]
      dyn-events: _ -> [_ _]
      timeout: w1235 -> [_ _]
      tunnel: w1234 -> [_ w1245]
      event Timeout {
        n447 = event-data() -> ()  [unwired: 1 in, 3 out]
      }
      event "Jog Z": Value Change {
        n448 = event-data() -> ()  [unwired: 1 in, 1 out]
        n449 = property on="Steps /um" class="DigNum (strict)"() -> ("Value"=w1244:dbl)  [unwired: 2 in, 2 out]
        n450 = Multiply(x=w1244, y=10.0) -> (x*y=w1247:dbl)
        n451 = Format Into String(format string="movrel\\sz=%f\\s\\r\\n", w1247) -> (resulting string=w1248:string)  [unwired: 2 in, 1 out]
        n452 = VISA Write(VISA resource name=w1245, write buffer=w1248) -> ()  [unwired: 1 in, 3 out]
      }
    }
    n453 = event shown="[2] \"405 power\": Mouse Up" {
      selector: _ -> [_ _ _]
      dyn-events: _ -> [_ _ _]
      timeout: w1235 -> [_ _ _]
      tunnel: w1233 -> [_ w1296 w1307]
      event Timeout {
        n454 = event-data() -> ()  [unwired: 1 in, 3 out]
      }
      event "405": Value Change {
        n455 = event-data() -> ("NewVal"=w1297:bool)  [unwired: 1 in, 5 out]
        n456 = case shown="False" w1297 {
          tunnel: w1296 -> [w1298 w1301]
          frame False {
            n457 = VISA Write(VISA resource name=w1298, write buffer="L 0\r\n" ("format string")) -> ()  [unwired: 1 in, 3 out]
          }
          frame True {
            n458 = VISA Write(VISA resource name=w1301, write buffer="L 1\r\n" ("format string")) -> ()  [unwired: 1 in, 3 out]
          }
        }
      }
      event "405 power": Mouse Up {
        n459 = event-data() -> ()  [unwired: 1 in, 8 out]
        n460 = Divide(x="405 power", y=100) -> (x/y=w1306:dbl)
        n461 = Multiply(x=w1306, y=110) -> (x*y=w1302:dbl)
        n462 = To Unsigned Byte Integer(number=w1302) -> (unsigned 8bit integer=w1310:u8)
        n463 = Number To Decimal String(number=w1310) -> (decimal integer string=w1311:string)  [unwired: 1 in]
        n464 = Concatenate Strings("PM ", w1311, "\r\n") -> (w1312:string)
        n465 = VISA Write(VISA resource name=w1307, write buffer=w1312) -> ()  [unwired: 1 in, 3 out]
      }
    }
    n466 = event shown="[2] \"488 power\": Mouse Up" {
      selector: _ -> [_ _ _]
      dyn-events: _ -> [_ _ _]
      timeout: w1235 -> [_ _ _]
      tunnel: w1242 -> [_ w1274 _]
      tunnel: w1236 -> [_ _ w1279]
      event Timeout {
        n467 = event-data() -> ()  [unwired: 1 in, 3 out]
      }
      event "488": Value Change {
        n468 = event-data() -> ("NewVal"=w1275:bool)  [unwired: 1 in, 5 out]
        n469 = call-poly <vilib>:"DAQmx Write.vi"("task/channels in"=w1274, "data"=w1275) -> ()  [unwired: 11 in, 3 out]
      }
      event "488 power": Mouse Up {
        n470 = event-data() -> ()  [unwired: 1 in, 1 out]
        n471 = Divide(x="488 power", y=200.0) -> (x/y=w1276:dbl)
        n472 = stacked-sequence {
          seq-local: [w1280 _ _ _] -> [_ _ w1292 _]
          seq-local: [_ _ w1291 _] -> [_ _ _ w1294]
          tunnel: w1276 -> [w1281 _ _ _]
          tunnel: w1279 -> [_ w1286 _ w1295]
          frame #0 {
            w1285 = "p"  # Command
            n473 = Number To Fractional String(use system decimal point (T)=FALSE, number=w1281) -> (F-format string=w1283:string)  [unwired: 2 in]
            n474 = call <vilib>:"Space Constant.vi"() -> ("String"=w1284:string)
            n475 = Concatenate Strings(w1285, w1284, w1283) -> (w1280:string)
          }
          frame #1 {
            n476 = VISA Flush I/O Buffer(VISA resource name=w1286, mask (16)=u16 128) -> (VISA resource name out=w1289:refnum<visa-resource-name>, error out=w1290:errorcluster)  [unwired: 1 in]
            n477 = VISA Flush I/O Buffer(VISA resource name=w1289, mask (16)=u16 64, error in (no error)=w1290) -> ()  [unwired: 2 out]
          }
          frame #2 {
            w1293 = "\r"  # StopChar
            n478 = Concatenate Strings(w1292, w1293) -> (w1291:string)
          }
          frame #3 {
            n479 = VISA Write(VISA resource name=w1295, write buffer=w1294) -> ()  [unwired: 1 in, 3 out]
          }
        }
      }
    }
    n480 = event shown="[0] Timeout" {
      selector: _ -> [_ _]
      dyn-events: _ -> [_ _]
      timeout: w1235 -> [_ _]
      tunnel: w1243 -> [_ w1272]
      event Timeout {
        n481 = event-data() -> ()  [unwired: 1 in, 3 out]
      }
      event "561": Value Change {
        n482 = event-data() -> ("NewVal"=w1273:bool)  [unwired: 1 in, 5 out]
        n483 = call-poly <vilib>:"DAQmx Write.vi"("task/channels in"=w1272, "data"=w1273) -> ()  [unwired: 11 in, 3 out]
      }
    }
    n484 = event shown="[1] \"647\": Value Change" {
      selector: _ -> [_ _ _]
      dyn-events: _ -> [_ _ _]
      timeout: w1235 -> [_ _ _]
      tunnel: w1238 -> [w1250 w1253 w1267]
      tunnel: [_ w1252 w1264] -> w1239
      tunnel: [w1250 w1251 w1265] -> w1240
      event Timeout {
        n485 = event-data() -> ()  [unwired: 1 in, 3 out]
      }
      event "647": Value Change {
        n486 = event-data() -> ("NewVal"=w1254:bool)  [unwired: 1 in, 5 out]
        n487 = case shown="True" w1254 {
          tunnel: w1253 -> [w1256 w1261]
          tunnel: [w1257 w1260] -> w1252
          tunnel: [w1255 w1259] -> w1251
          frame False {
            n488 = VISA Write(VISA resource name=w1256, write buffer="la off\r" ("format string")) -> (VISA resource name out=w1255:refnum<visa-resource-name>, error out=w1257:errorcluster)  [unwired: 1 in, 1 out]
          }
          frame True {
            n489 = VISA Write(VISA resource name=w1261, write buffer="la on\r" ("format string")) -> (VISA resource name out=w1259:refnum<visa-resource-name>, error out=w1260:errorcluster)  [unwired: 1 in, 1 out]
          }
        }
      }
      event "647 Power": Mouse Up {
        n490 = event-data() -> ()  [unwired: 1 in, 1 out]
        n491 = To Unsigned Byte Integer(number="647 Power") -> (unsigned 8bit integer=w1271:u8)
        n492 = Number To Decimal String(number=w1271) -> (decimal integer string=w1269:string)  [unwired: 1 in]
        n493 = Concatenate Strings("ch 1 pow ", w1269, "\r") -> (w1266:string)
        n494 = VISA Write(VISA resource name=w1267, write buffer=w1266) -> (VISA resource name out=w1265:refnum<visa-resource-name>, error out=w1264:errorcluster)  [unwired: 1 in, 1 out]
      }
    }
    n495 = property on="stop" class="Bool (strict)"() -> ("Value"=w1241:bool)  [unwired: 2 in, 2 out]
  }
  n496 = while {
    tunnel: w31 -> [w1323]
    tunnel: w32 -> [w1322]
    tunnel: w27 -> [w1324]
    tunnel: ["stop"] -> _
    tunnel: [w1324] -> w89
    tunnel: [w1323] -> w88
    tunnel: [w1322] -> w90
    shift-right: [w1316] -> _
    shift-left: 0 -> [w1315]
    tunnel: w39 -> [w1313]
    tunnel: [w1313] -> w38
    stop <- "stop" stop-if-true
    n497 = Greater?(x=w1315, y=8) -> (0:w1318:bool)
    n498 = Select(t=0, s=w1318, f=w1315) -> (s? t:f=w1317:i32)
    n499 = Add(x=1, y=w1317) -> (x+y=w1316:i32)
    "x+y" <- w1316
    n500 = case shown="True" "Go live" {
      tunnel: w1324 -> [_ w1331]
      tunnel: w1323 -> [_ w1330]
      tunnel: w1322 -> [_ w1329]
      tunnel: w1316 -> [_ w1326]
      frame False {
      }
      frame True {
        n501 = property on="561 voltages" class="Arr (strict)"() -> ("Value"=w1327:dbl[][])  [unwired: 2 in, 2 out]
        n502 = case shown="\"Static\", Default" "Live mode" {
          tunnel: w1327 -> [_ w1382 w1432 w1470]
          tunnel: w1330 -> [_ w1379 w1418 w1464]
          tunnel: w1329 -> [w1333 w1365 w1420 _]
          tunnel: w1331 -> [w1332 w1366 w1419 _]
          tunnel: w1326 -> [_ _ w1408 _]
          frame "Static", Default {
            n503 = flat-sequence {
              tunnel: w1333 -> [w1346]
              tunnel: [w1344] -> w1341
              tunnel: [w1343] -> w1340
              tunnel: w1332 -> [w1342]
              tunnel: [w1342] -> w1339
              tunnel: w1341 -> [w1350]
              tunnel: [w1350] -> w1338
              tunnel: w1340 -> [w1348]
              tunnel: [w1349] -> w1337
              tunnel: w1339 -> [w1349]
              tunnel: [w1348] -> w1336
              tunnel: w1338 -> [w1355]
              tunnel: [w1353] -> w1335
              tunnel: w1337 -> [w1353]
              tunnel: w1336 -> [w1352]
              tunnel: [w1351] -> w1334
              tunnel: w1335 -> [w1358]
              tunnel: w1334 -> [w1357]
              tunnel: [w1356] -> _
              frame #0 {
                n504 = call-poly <vilib>:"DAQmx Write.vi"("task/channels in"=w1346, "data"=TRUE) -> ("task out"=w1344:refnum<k21>, "error out"=w1343:errorcluster)  [unwired: 11 in, 1 out]
              }
              frame #1 {
                n505 = property on="Exposure time" class="DigNum (strict)"() -> ("Value"=w1347:dbl)  [unwired: 2 in, 2 out]
                n506 = Wait (ms)(milliseconds to wait=w1347) -> ()  [unwired: 1 out]
              }
              frame #2 {
                n507 = call-poly <vilib>:"DAQmx Write.vi"("task/channels in"=w1355, "data"=FALSE, "error in"=w1352) -> ("error out"=w1351:errorcluster)  [unwired: 10 in, 2 out]
              }
              frame #3 {
                n508 = while {
                  tunnel: w1358 -> [w1363]
                  tunnel: w1357 -> [w1362]
                  tunnel: [w1361] -> w1356
                  stop <- w1360 stop-if-true
                  n509 = call-poly <vilib>:"DAQmx Read.vi"("task/channels in"=w1363, "error in"=w1362) -> ("data"=w1359:bool, "error out"=w1361:errorcluster)  [unwired: 11 in, 1 out]
                  n510 = Not(x=w1359) -> (.not. x?=w1360:bool)
                }
              }
            }
          }
          frame "Widefield" {
            n511 = Index Array(array=w1382, index (row)=2, index (col)=1) -> ()  [unwired: 1 out]
            n512 = call <vilib>:"Triangle Waveform.vi"("offset"=1.0, "phase"=0.0, "amplitude"=0.06, "frequency"=0.1) -> ("signal out"=w1375:waveform(dbl))  [unwired: 6 in, 1 out]
            n513 = call-poly <vilib>:"DAQmx Write.vi"("task/channels in"=w1379, "data"=w1375) -> ()  [unwired: 11 in, 3 out]
            n514 = flat-sequence {
              tunnel: w1365 -> [w1387]
              tunnel: [w1385] -> w1374
              tunnel: [w1384] -> w1373
              tunnel: [w1383] -> w1372
              tunnel: w1366 -> [w1383]
              tunnel: w1374 -> [w1391]
              tunnel: [w1391] -> w1371
              tunnel: w1373 -> [w1389]
              tunnel: [w1390] -> w1370
              tunnel: w1372 -> [w1390]
              tunnel: [w1389] -> w1369
              tunnel: w1371 -> [w1396]
              tunnel: [w1394] -> w1368
              tunnel: w1370 -> [w1394]
              tunnel: w1369 -> [w1393]
              tunnel: [w1392] -> w1367
              tunnel: w1368 -> [w1399]
              tunnel: w1367 -> [w1398]
              tunnel: [w1397] -> _
              frame #0 {
                n515 = call-poly <vilib>:"DAQmx Write.vi"("task/channels in"=w1387, "data"=TRUE) -> ("task out"=w1385:refnum<k21>, "error out"=w1384:errorcluster)  [unwired: 11 in, 1 out]
              }
              frame #1 {
                n516 = property on="Exposure time" class="DigNum (strict)"() -> ("Value"=w1388:dbl)  [unwired: 2 in, 2 out]
                n517 = Wait (ms)(milliseconds to wait=w1388) -> ()  [unwired: 1 out]
              }
              frame #2 {
                n518 = call-poly <vilib>:"DAQmx Write.vi"("task/channels in"=w1396, "data"=FALSE, "error in"=w1393) -> ("error out"=w1392:errorcluster)  [unwired: 10 in, 2 out]
              }
              frame #3 {
                n519 = while {
                  tunnel: w1399 -> [w1404]
                  tunnel: w1398 -> [w1403]
                  tunnel: [w1402] -> w1397
                  stop <- w1401 stop-if-true
                  n520 = call-poly <vilib>:"DAQmx Read.vi"("task/channels in"=w1404, "error in"=w1403) -> ("data"=w1400:bool, "error out"=w1402:errorcluster)  [unwired: 11 in, 1 out]
                  n521 = Not(x=w1400) -> (.not. x?=w1401:bool)
                }
              }
            }
          }
          frame "SIM" {
            n522 = Quotient & Remainder(x=w1408, y=9) -> (x-y*floor(x/y)=w1430:i32)  [unwired: 1 out]
            n523 = flat-sequence {
              tunnel: w1419 -> [w1436]
              tunnel: w1420 -> [w1437]
              tunnel: [w1437] -> w1417
              tunnel: [w1433] -> w1415
              tunnel: [w1436] -> w1413
              tunnel: w1418 -> [w1435]
              tunnel: w1407 -> [w1434]
              tunnel: w1417 -> [w1441]
              tunnel: [w1441] -> w1416
              tunnel: w1415 -> [w1440]
              tunnel: [w1440] -> w1414
              tunnel: w1413 -> [w1439]
              tunnel: [w1439] -> w1412
              tunnel: [w1445] -> w1428
              tunnel: [w1443] -> w1427
              tunnel: [w1442] -> w1426
              tunnel: w1416 -> [w1447]
              tunnel: w1414 -> [w1444]
              tunnel: w1412 -> [w1442]
              tunnel: w1428 -> [w1451]
              tunnel: [w1451] -> w1425
              tunnel: w1427 -> [w1449]
              tunnel: [w1450] -> w1424
              tunnel: w1426 -> [w1450]
              tunnel: [w1449] -> w1423
              tunnel: w1425 -> [w1456]
              tunnel: [w1454] -> w1422
              tunnel: w1424 -> [w1454]
              tunnel: w1423 -> [w1453]
              tunnel: [w1452] -> w1421
              tunnel: w1422 -> [w1458]
              tunnel: w1421 -> [w1457]
              frame #0 {
                n524 = call-poly <vilib>:"DAQmx Write.vi"("task/channels in"=w1435, "data"=w1434) -> ("error out"=w1433:errorcluster)  [unwired: 11 in, 2 out]
              }
              frame #1 {
                n525 = property on="Settle time" class="DigNum (strict)"() -> ("Value"=w1438:u32)  [unwired: 2 in, 2 out]
                n526 = Wait (ms)(milliseconds to wait=w1438) -> ()  [unwired: 1 out]
              }
              frame #2 {
                n527 = call-poly <vilib>:"DAQmx Write.vi"("task/channels in"=w1447, "data"=TRUE, "error in"=w1444) -> ("task out"=w1445:refnum<k21>, "error out"=w1443:errorcluster)  [unwired: 10 in, 1 out]
              }
              frame #3 {
                n528 = property on="Exposure time" class="DigNum (strict)"() -> ("Value"=w1448:dbl)  [unwired: 2 in, 2 out]
                n529 = Wait (ms)(milliseconds to wait=w1448) -> ()  [unwired: 1 out]
              }
              frame #4 {
                n530 = call-poly <vilib>:"DAQmx Write.vi"("task/channels in"=w1456, "data"=FALSE, "error in"=w1453) -> ("error out"=w1452:errorcluster)  [unwired: 10 in, 2 out]
              }
              frame #5 {
                n531 = while {
                  tunnel: w1458 -> [w1463]
                  tunnel: w1457 -> [w1462]
                  tunnel: [w1461] -> _
                  stop <- w1460 stop-if-true
                  n532 = call-poly <vilib>:"DAQmx Read.vi"("task/channels in"=w1463, "error in"=w1462) -> ("data"=w1459:bool, "error out"=w1461:errorcluster)  [unwired: 11 in, 1 out]
                  n533 = Not(x=w1459) -> (.not. x?=w1460:bool)
                }
              }
            }
            n534 = Add(x=0, y=w1430) -> (x+y=w1409:i32)
            n535 = Index Array(array=i32[] [1, 2, 0, 1, 2, 0, 1, 2, 0, 0, 1, 2, 3, 4, 0], index=w1409) -> (element=w1405:i32)
            n536 = Index Array(array=i32[] [0, 0, 1, 1, 1, 2, 2, 2, 0, 2, 2, 2, 2, 2, 0], index=w1409) -> (element=w1406:i32)
            n537 = Index Array(array=w1432, index (row)=w1405, index (col)=w1406) -> (element=w1407:dbl)
            n538 = property on="Current voltage" class="DigNum (strict)"("Value"=w1407) -> ()  [unwired: 2 in, 2 out]
          }
          frame "Strobe" {
            n539 = flat-sequence {
              tunnel: w1470 -> [w1472]
              tunnel: [w1472] -> w1468
              tunnel: w1464 -> [w1471]
              tunnel: [w1477] -> w1469
              tunnel: w1468 -> [w1477]
              tunnel: w1469 -> [w1479]
              tunnel: [w1479] -> w1467
              tunnel: w1464 -> [w1478]
              tunnel: w1467 -> [w1484]
              tunnel: [w1484] -> w1466
              tunnel: w1466 -> [w1486]
              tunnel: [w1486] -> w1465
              tunnel: w1464 -> [w1485]
              tunnel: [w1491] -> _
              tunnel: w1465 -> [w1491]
              frame #0 {
                n540 = Index Array(array=w1472, index (row)=2, index (col)=0) -> (element=w1473:dbl)
                n541 = call-poly <vilib>:"DAQmx Write.vi"("task/channels in"=w1471, "data"=w1473) -> ()  [unwired: 11 in, 3 out]
              }
              frame #1 {
                n542 = property on="Settle time" class="DigNum (strict)"() -> ("Value"=w1476:u32)  [unwired: 2 in, 2 out]
                n543 = Wait (ms)(milliseconds to wait=w1476) -> ()  [unwired: 1 out]
              }
              frame #2 {
                n544 = Index Array(array=w1479, index (row)=2, index (col)=1) -> (element=w1482:dbl)
                n545 = call-poly <vilib>:"DAQmx Write.vi"("task/channels in"=w1478, "data"=w1482) -> ()  [unwired: 11 in, 3 out]
              }
              frame #3 {
                n546 = property on="Settle time" class="DigNum (strict)"() -> ("Value"=w1483:u32)  [unwired: 2 in, 2 out]
                n547 = Wait (ms)(milliseconds to wait=w1483) -> ()  [unwired: 1 out]
              }
              frame #4 {
                n548 = Index Array(array=w1486, index (row)=2, index (col)=2) -> (element=w1487:dbl)
                n549 = call-poly <vilib>:"DAQmx Write.vi"("task/channels in"=w1485, "data"=w1487) -> ()  [unwired: 11 in, 3 out]
              }
              frame #5 {
                n550 = property on="Settle time" class="DigNum (strict)"() -> ("Value"=w1490:u32)  [unwired: 2 in, 2 out]
                n551 = Wait (ms)(milliseconds to wait=w1490) -> ()  [unwired: 1 out]
              }
            }
          }
        }
      }
    }
    "?" <- "Go live"
  }
  n552 = VISA Write(VISA resource name=w13, write buffer="L 0\n" ("format string")) -> (VISA resource name out=w12:refnum<visa-resource-name>)  [unwired: 1 in, 2 out]
  n553 = call-poly <vilib>:"DAQmx Write.vi"("task/channels in"=w81, "data"=w79) -> ("task out"=w75:refnum<k21>, "error out"=w73:errorcluster)  [unwired: 11 in, 1 out]
  n554 = call-poly <vilib>:"DAQmx Write.vi"("task/channels in"=w80, "data"=w79) -> ("task out"=w76:refnum<k21>, "error out"=w74:errorcluster)  [unwired: 11 in, 1 out]
  n555 = call <vilib>:"DAQmx Stop Task.vi"("task/channels in"=w38) -> ("task out"=w37:refnum<k21>)  [unwired: 13 in, 1 out]
  n556 = call <vilib>:"DAQmx Stop Task.vi"("task/channels in"=w75, "error in"=w73) -> ("task out"=w78:refnum<k21>, "error out"=w72:errorcluster)  [unwired: 12 in]
  n557 = call <vilib>:"DAQmx Stop Task.vi"("task/channels in"=w76, "error in"=w74) -> ("task out"=w77:refnum<k21>, "error out"=w71:errorcluster)  [unwired: 12 in]
  n558 = call <vilib>:"DAQmx Clear Task.vi"("task in"=w37) -> ("error out"=w36:errorcluster)  [unwired: 14 in]
  n559 = VISA Write(VISA resource name=w10, write buffer="la off\r" ("format string")) -> (VISA resource name out=w9:refnum<visa-resource-name>)  [unwired: 1 in, 2 out]
  n560 = call <vilib>:"DAQmx Stop Task.vi"("task/channels in"=w90) -> ("task out"=w85:refnum<k21>)  [unwired: 13 in, 1 out]
  n561 = call <vilib>:"DAQmx Stop Task.vi"("task/channels in"=w88) -> ("task out"=w87:refnum<k21>)  [unwired: 13 in, 1 out]
  n562 = call <vilib>:"DAQmx Stop Task.vi"("task/channels in"=w89) -> ("task out"=w86:refnum<k21>)  [unwired: 13 in, 1 out]
  n563 = call <vilib>:"DAQmx Clear Task.vi"("task in"=w85) -> ("error out"=w50:errorcluster)  [unwired: 14 in]
  n564 = call <vilib>:"DAQmx Clear Task.vi"("task in"=w78, "error in"=w72) -> ("error out"=w69:errorcluster)  [unwired: 13 in]
  n565 = call <vilib>:"DAQmx Clear Task.vi"("task in"=w77, "error in"=w71) -> ("error out"=w70:errorcluster)  [unwired: 13 in]
  n566 = VISA Close(VISA resource name=w61, error in (no error)=w60) -> (error out=w59:errorcluster)
  n567 = VISA Close(VISA resource name=w9) -> (error out=w28:errorcluster)  [unwired: 1 in]
  n568 = VISA Close(VISA resource name=w12) -> (error out=w15:errorcluster)  [unwired: 1 in]
  n569 = call <vilib>:"DAQmx Clear Task.vi"("task in"=w87) -> ("error out"=w83:errorcluster)  [unwired: 14 in]
  n570 = Merge Errors(w69, w70, w59, w28, w15) -> (→"Laser error":errorcluster)
  n571 = call <vilib>:"DAQmx Clear Task.vi"("task in"=w86) -> ("error out"=w82:errorcluster)  [unwired: 14 in]
  n572 = property on="Go live" class="Bool (strict)"(error in=w50, "Value"=FALSE) -> (error out=w49:errorcluster)  [unwired: 1 in, 1 out]
  n573 = Merge Errors(w83, w82, w49, w36) -> (→"Camera/galvo error":errorcluster)
  n574 = VISA Close(VISA resource name=w67) -> ()  [unwired: 1 in, 1 out]
